vi "Turbo Process Mngr.vi"(0 "State In":T1, 1 "Mngr Action":T12, 2 "FP":T11, 7 "Cartridges":T5, 9 "Manual Input":dbl format="%#_13g", 11 "error in (no error)":errorcluster, 12 "Config":T2={"Syringe size"=0, "Syringe address"=0, "# of ports"=0, "Init String"="Z0N1R", "Full Stroke (cnts)"=0, "Model"=enum."XC", "TW Position"=0.0, "Load Position"=0.0, "Bottom Position"=0.0, "Station ID"="", "Default Protocol"=path "", "Dry Time(s)"=0.0, "Python Version"="", "NFC SN Array"=["21121521200223", "21121521200186", "21121521200213", "52541737200062"], "Timing"={"Checking pres and leak"=0.0, "Priming input lines"=0.0, "Rinsing syringe"=0.0, "Filling well X w/ X"=0.0, "Drain well X"=0.0, "Clearing wells and lines"=0.0, "Draining wells"=0.0, "Rinsing all wells"=0.0, "Testing for leaks/clogs"=0.0, "Rinsing wells"=0.0}, "Pressure Specs"={"Pressure max"=0.0, "Pressure min"=0.0, "Decay delta"=0.0, "Pressure time"=0.0, "Conf. R"=0.0, "LeakRateMax"=0.0}}) -> (15 "error out":errorcluster)   [LabVIEW 2020]
uses:
  Process Mngr.ctl
  Main Refs.ctl
  Wash Step.ctl
  Results.ctl
  Vacuum Test.ctl
  Pressure Output.ctl
  Process Turbo.ctl
  Cartridge #.ctl
  Hardware/Tecan/Pump Config.ctl
  Timing Specs.ctl
  Vacuum Specs.ctl
  status update.ctl
  Cartridge Mngr.ctl
  Time elapsed.ctl
  Hardware/DAQ Mngr.ctl
  Hardware/Mot Stage Mngr.ctl
  Update Single Cart.ctl
  Lib/Time/Bottles.ctl
  Hardware/16CH Denkovi Mngr.ctl
  Hardware/Tricon Mngr.ctl
  Hardware/Tecan/Pump Control.ctl
  Pump Port.ctl
  Hardware/Tecan/Velocity Units.ctl
  Main Globals.vi
  Lib/Utilities.lvlib
panel:
  out "State Out":T1
  out "Wash Time(s) 2":dbl
  out "Wash Time(s)":dbl
  out "Reports":T6[](array[typedef])
  in  "Pressure Specs":T9
  out "Wash Array":T10[](array[typedef]) {"# of Rinses" max=10}
  # "Tecan Pump"
  # "Pressure"
  # "General"
  # "Timing"
  # "Protocol"
  # "Zaber"
  # "NFC Reader 1"
  # "NFC  Reader 2"
  # "NFC Reader 3"
  # "NFC Reader 4"
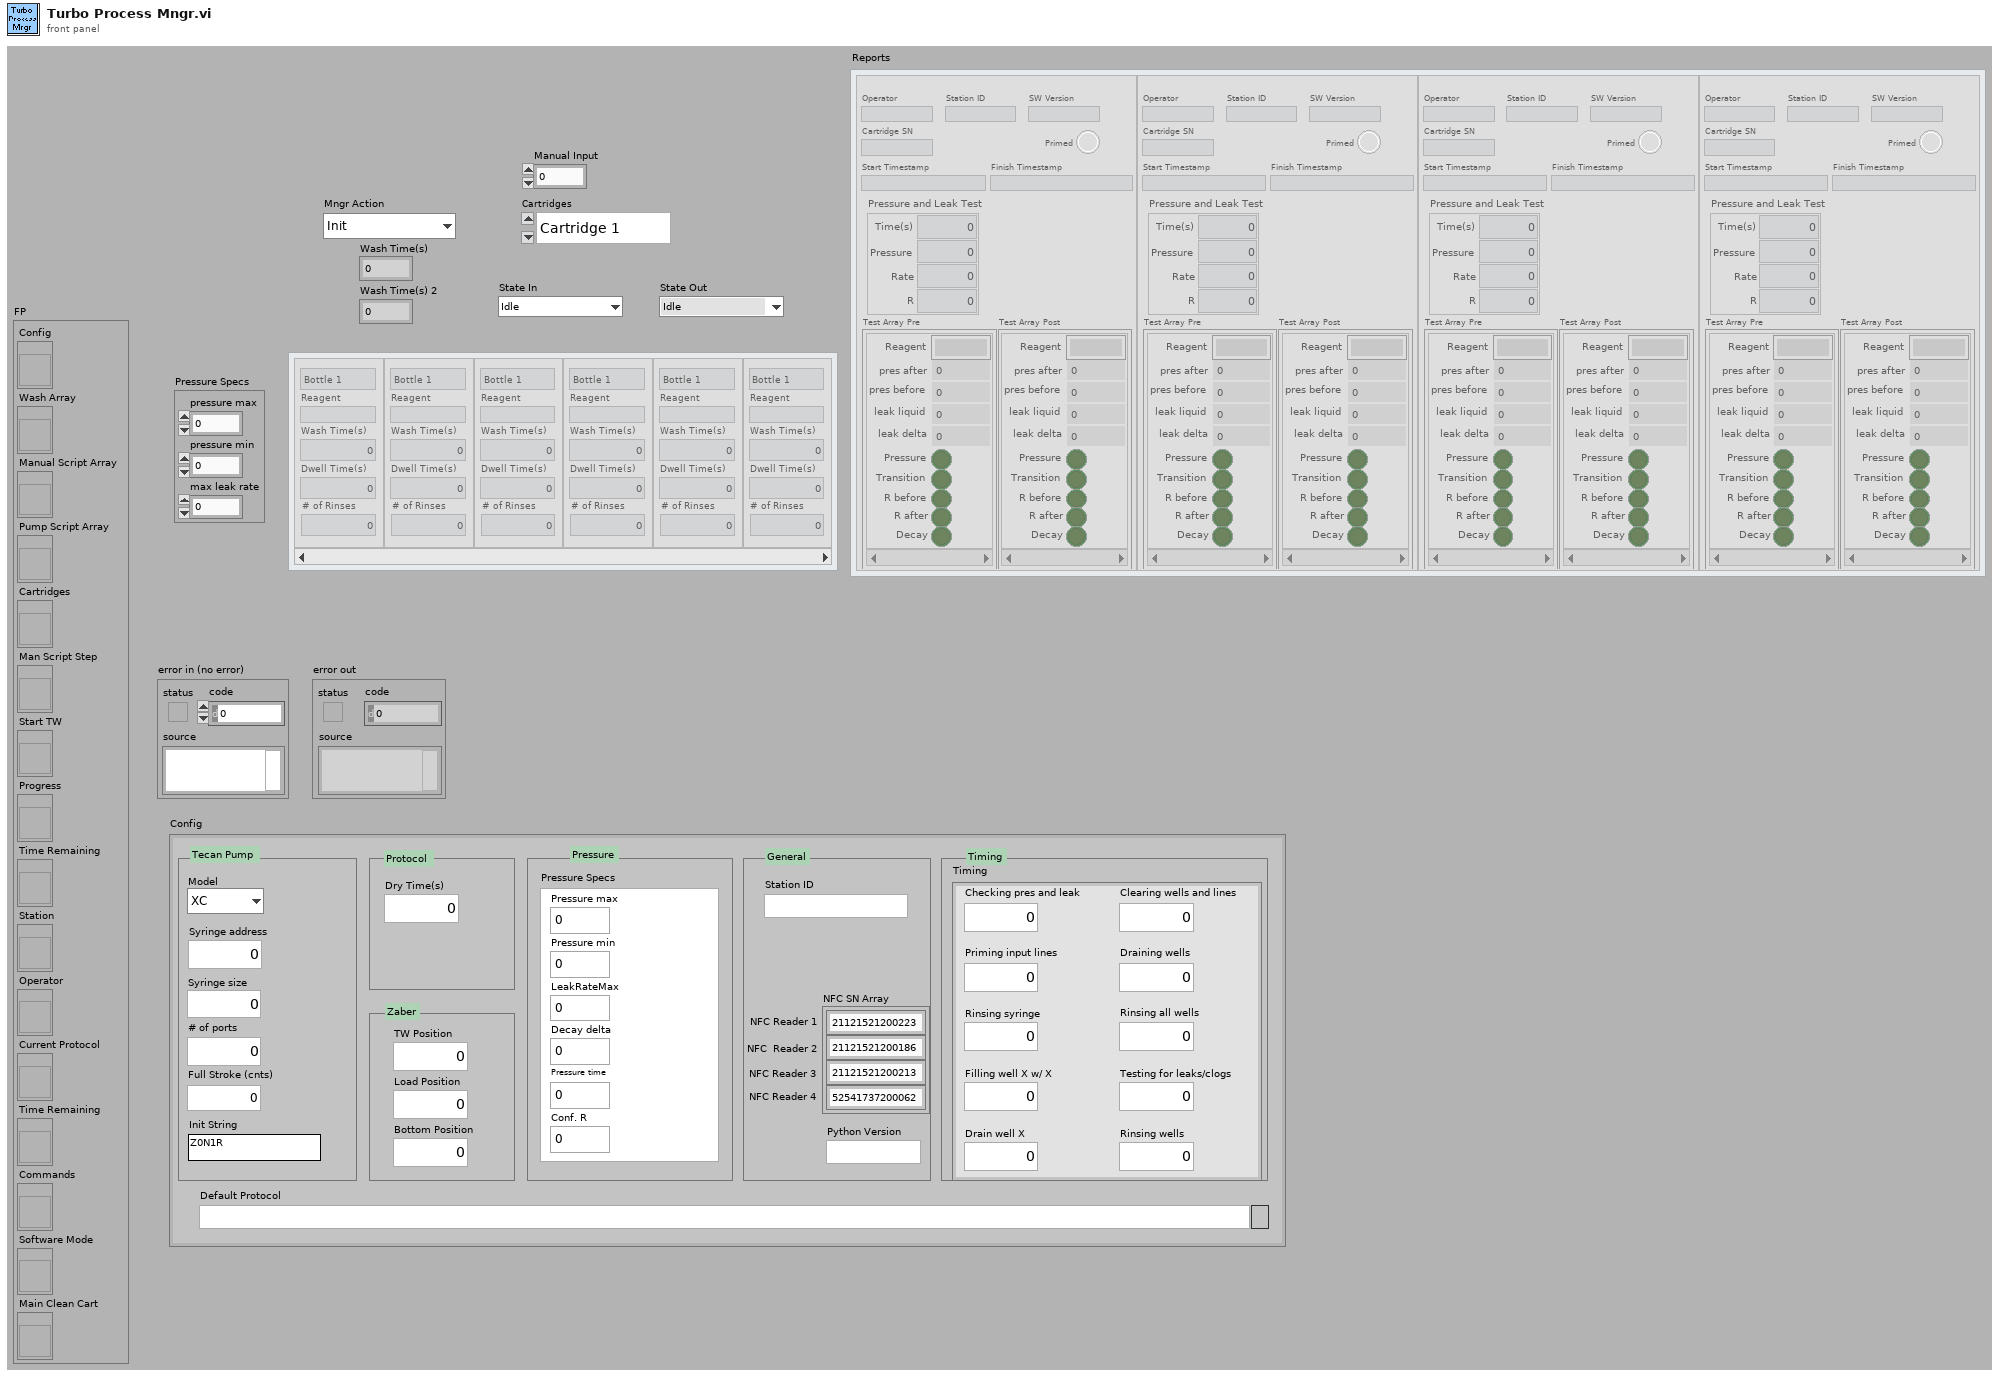
[diagram p1: front panel]
types:
  T1 = typedef "Process Turbo.ctl" = enum16{"Idle", "Init", "Check for SN", "Start TW", "SystemLeakTest", "Prime System", "Rinse Wells", "Fill Wells", "High Vac On", "Pressure&Vac Load", "Trap Vac", "PrePresTest", "Apply Pressure", "PostPresTest", "Drain&Rinse", "Dry", "Report", "Finish", "Abort", "Error", "-rinse wells", "-check cartridge", "-clean cartridge", "-drain all", "-fill well"}
  T2 = typedef "Pump Config.ctl" = cluster{"Syringe size":u32, "Syringe address":u32, "# of ports":u32, "Init String":string, "Full Stroke (cnts)":i32, "Model":enum16{"XC", "Centris"}, "TW Position":dbl, "Load Position":dbl, "Bottom Position":dbl, "Station ID":string, "Default Protocol":path, "Dry Time(s)":dbl, "Python Version":string, "NFC SN Array":string[], "Timing":T3, "Pressure Specs":T4}
  T3 = typedef "Timing Specs.ctl" = cluster{"Checking pres and leak":dbl, "Priming input lines":dbl, "Rinsing syringe":dbl, "Filling well X w/ X":dbl, "Drain well X":dbl, "Clearing wells and lines":dbl, "Draining wells":dbl, "Rinsing all wells":dbl, "Testing for leaks/clogs":dbl, "Rinsing wells":dbl}
  T4 = typedef "Vacuum Specs.ctl" = cluster{"Pressure max":dbl, "Pressure min":dbl, "Decay delta":dbl, "Pressure time":dbl, "Conf. R":dbl, "LeakRateMax":dbl}
  T5 = typedef "Cartridge #.ctl" = enum16{"Cartridge 1", "Cartridge 2", "Cartridge 3", "Cartridge 4"}
  T6 = typedef "Results.ctl" = cluster{"Operator":string, "Station ID":string, "SW Version":string, "Cartridge SN":string, "Primed":bool, "Start Timestamp":string, "Finish Timestamp":string, "Test Array Pre":T7[], "Test Array Post":T7[], "Pressure and Leak Test":T8}
  T7 = typedef "Vacuum Test.ctl" = cluster{"pres after":dbl, "pres before":dbl, "leak liquid":dbl, "leak delta":dbl, "Transition":bool, "Pressure":bool, "R before":bool, "R after":bool, "Reagent":string, "Decay":bool}
  T8 = typedef "Pressure Output.ctl" = cluster{"Time(s)":dbl, "Pressure":dbl, "Rate":dbl, "R":dbl}
  T9 = cluster{"pressure max":dbl, "pressure min":dbl, "max leak rate":dbl}
  T10 = typedef "Wash Step.ctl" = cluster{"Reagent":string, "Bottle":enum16{"Bottle 1", "Bottle 2", "Bottle 3", "Bottle 4"}, "Wash Time(s)":dbl, "Dwell Time(s)":dbl, "# of Rinses":i16}
  T11 = typedef "Main Refs.ctl" = cluster{"Config":refnum<vi>, "Wash Array":refnum<vi>, "Manual Script Array":refnum<vi>, "Pump Script Array":refnum<vi>, "Cartridges":refnum<vi>, "Man Script Step":refnum<vi>, "Start TW":refnum<vi>, "Progress":refnum<vi>, "Time Remaining":refnum<vi>, "Station":refnum<vi>, "Operator":refnum<vi>, "Current Protocol":refnum<vi>, "Time Remaining":refnum<vi>, "Commands":refnum<vi>, "Software Mode":refnum<vi>, "Main Clean Cart":refnum<vi>}
  T12 = typedef "Process Mngr.ctl" = enum16{"Init", "Run Step", "Update"}
  T13 = enum8{"Enabled", "Disabled", "Disabled and Grayed Out"}
  T14 = typedef "status update.ctl" = enum16{"Cartridge", "Main Status", "Reagent"}
  T15 = typedef "Cartridge Mngr.ctl" = enum16{"Init", "Update", "Detect", "Lock", "Read SN", "Unlock", "Error"}
  T16 = enum16{"Init Pressure", "Init Vacuum", "Save Pressure", "Save Vacuum", "Close"}
  T17 = typedef "DAQ Mngr.ctl" = enum16{"Init", "Read Pressure", "Read Vacuum", "Analyze Pres&Vac", "Analyze Vacuum", "Read Cartridges", "Lock Cartridge", "Unlock Cartridge", "Read PS", "Pinch Valve Engage", "Pinch Valve Disengage", "Close"}
  T18 = typedef "Time elapsed.ctl" = enum16{"Start", "Update", "Read"}
  T19 = typedef "Mot Stage Mngr.ctl" = enum16{"Connect", "Init", "Status", "Send Cmd", "Current Pos", "Set Accel", "Set Max Vel", "Home", "Rel Move", "Abs Move", "Close"}
  T20 = typedef "Update Single Cart.ctl" = enum16{"Cart Status", "Cart Reagent"}
  T21 = typedef "Bottles.ctl" = enum16{"Bottle 1", "Bottle 2", "Bottle 3", "H2O", "Waste"}
  T22 = typedef "16CH Denkovi Mngr.ctl" = enum16{"Search", "Init", "Set Peristaltic", "Set Pressure", "Set Vacuum", "Set PresVac", "Pres Vent&Close", "Vac Vent&Close", "Pres ON", "Vac ON", "Set All Relays", "Set One Relay", "Read Relays", "Close"}
  T23 = typedef "Pump Control.ctl" = cluster{"Syringe Pos":u32, "Rate":dbl, "Volume":dbl, "Valve":T24, "Action":enum32{"Withdraw", "Dispense", "Stop"}, "Move Type":enum32{"Abs", "Rel"}, "Init":bool, "Empty Syr.":bool, "Full Fill":bool, "Units":T25}
  T24 = typedef "Pump Port.ctl" = enum16{"Bottle 1", "Bottle 2", "Bottle 3", "Bottle 4", "Waste", "Well 1", "Well 2", "Well 3", "Well 4", "Bottle X", "Well X"}
  T25 = typedef "Velocity Units.ctl" = enum16{"ul/s", "ul/min"}
  T26 = typedef "Tricon Mngr.ctl" = enum16{"Init COM", "Set Config", "Init Pump", "Home", "Cmd", "Start Pump", "Set Valve", "Dispense", "Withdraw", "Status", "Close"}
  T27 = typedef "Cartridges.ctl" = cluster{"Cartridge 1":T28, "Cartridge 2":T28, "Cartridge 3":T28, "Cartridge 4":T28, "Current Status":string}
  T28 = typedef "Cartridge Status.ctl" = cluster{"Serial Number":string, "Reagent":string, "Cart Status":string, "Inserted":bool, "Eject":bool}
  T29 = typedef "Vacuum Output.ctl" = cluster{"Time(s)":dbl, "Vacuum":dbl, "Rate":dbl, "R":dbl}
  T30 = enum16{"Bottle 1", "Bottle 2", "Bottle 3", "Bottle 4"}
  T31 = typedef "Commands.ctl" = cluster{"Drain All Wells":bool, "Rinse All Wells":bool, "Prime":bool, "Well #":T32, "Bottle #":T21, "Fill":bool, "Run State":bool, "State":T33, "Empty Lines":bool, "Clean&Dry Cartridge":bool, "Check for leaks":bool, "Cart Test Array":T7[], "Number of rinses":dbl}
  T32 = typedef "Wells.ctl" = enum16{"Well 1", "Well 2", "Well 3", "Well 4"}
  T33 = typedef "Process State.ctl" = enum16{"Idle", "Init", "Check for SN", "Start TW", "SystemLeakTest", "Prime System", "Rinse Wells", "Fill Wells", "PrePresTest", "Apply Pressure", "PostPresTest", "Drain&Rinse", "Dry", "Report", "Finish", "Abort", "Error", "-rinse wells", "-check cartridge", "-clean cartridge", "-drain all", "-fill well"}
  T34 = cluster{"negative limit switch":bool, "positive limit switch":bool, "home switch":bool, "position marker":bool, "device enable":bool, "quick stop":bool, "general purpose J":bool, "general purpose I":bool, "general purpose H":bool, "general purpose G":bool, "general purpose F":bool, "general purpose E":bool, "general purpose D":bool, "general purpose C":bool, "general purpose B":bool, "general purpose A":bool}
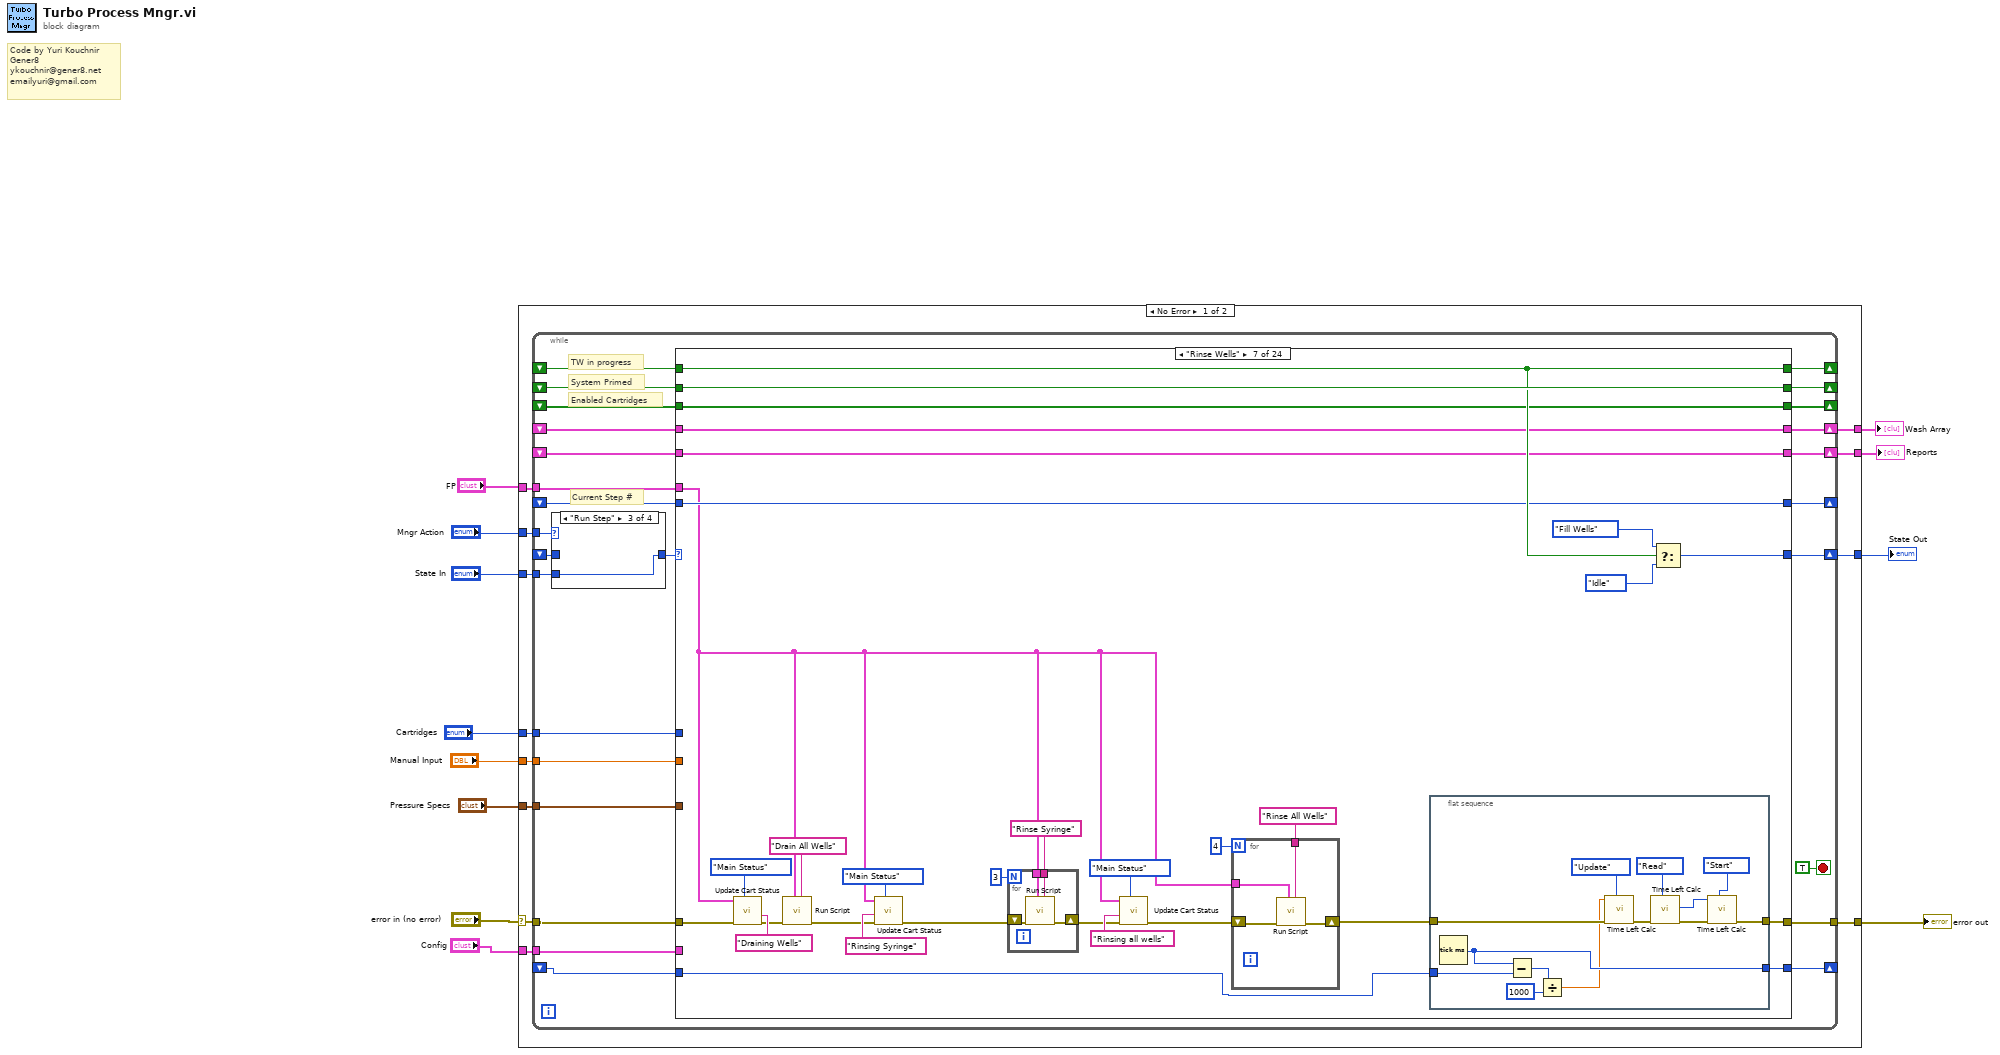
[diagram p0: block diagram]
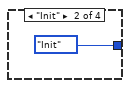
[diagram p3: hidden frame]
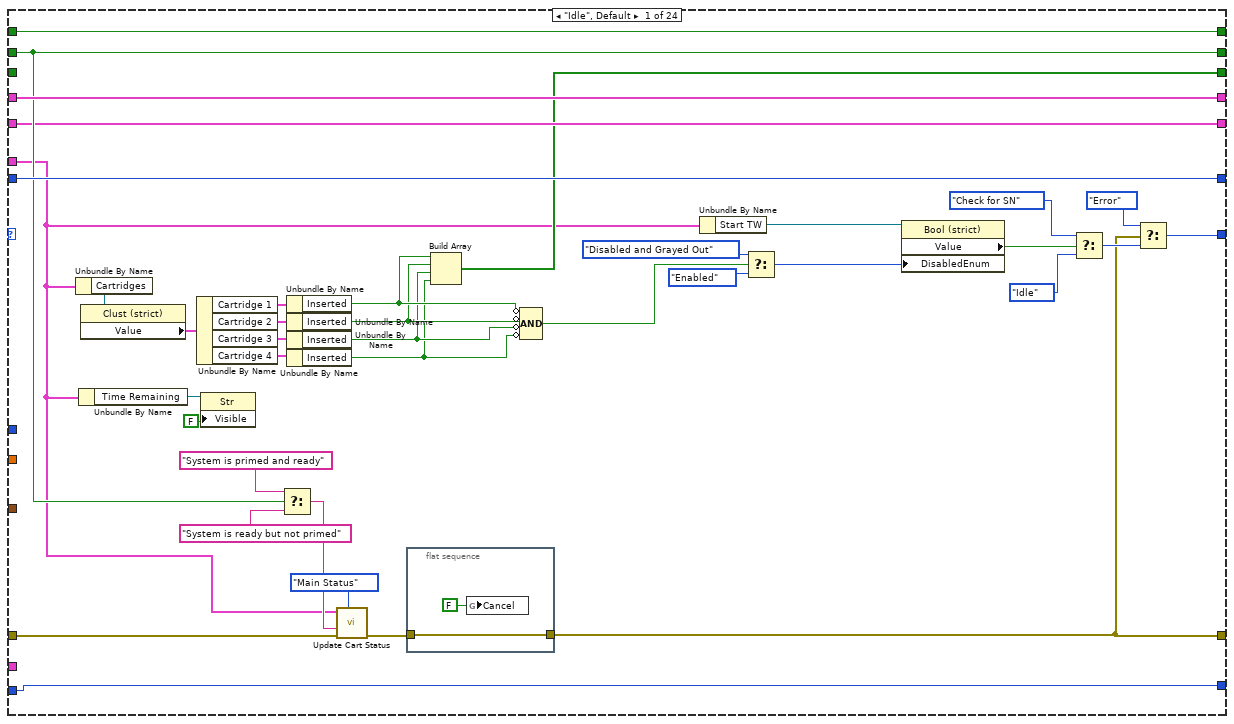
[diagram p5: hidden frame]
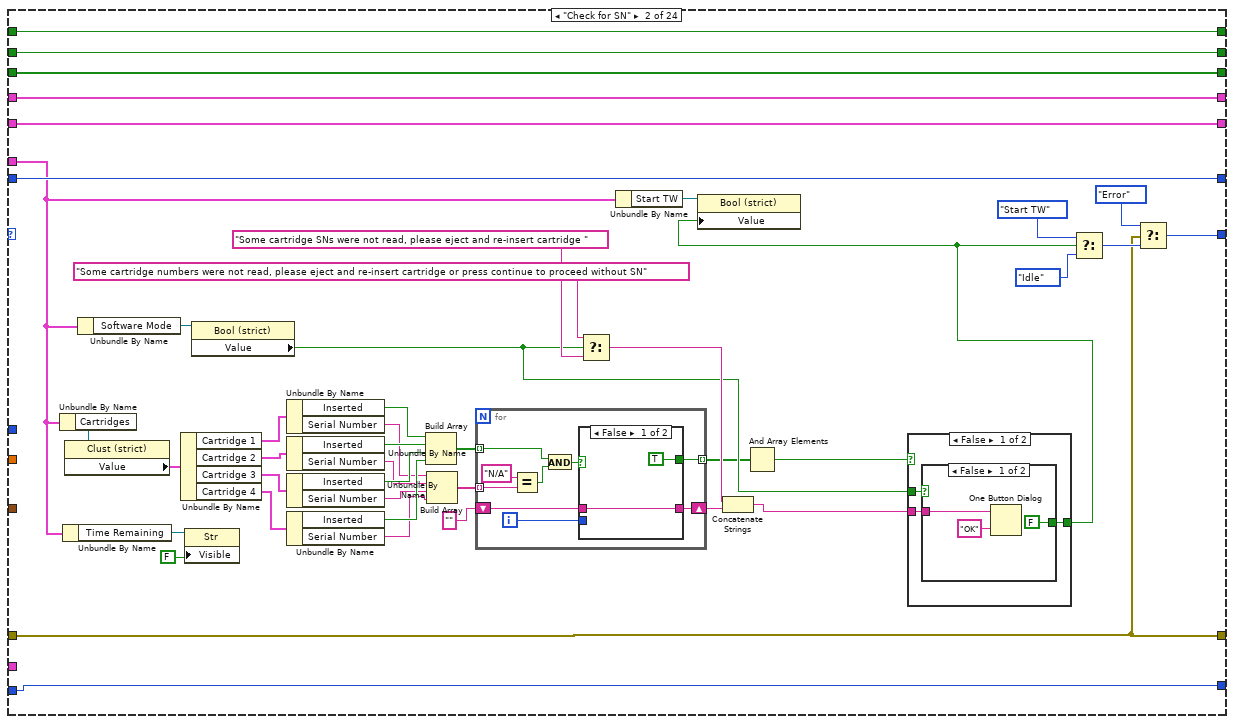
[diagram p6: hidden frame]
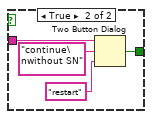
[diagram p7: hidden frame]
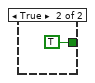
[diagram p8: hidden frame]
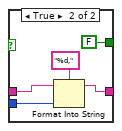
[diagram p9: hidden frame]
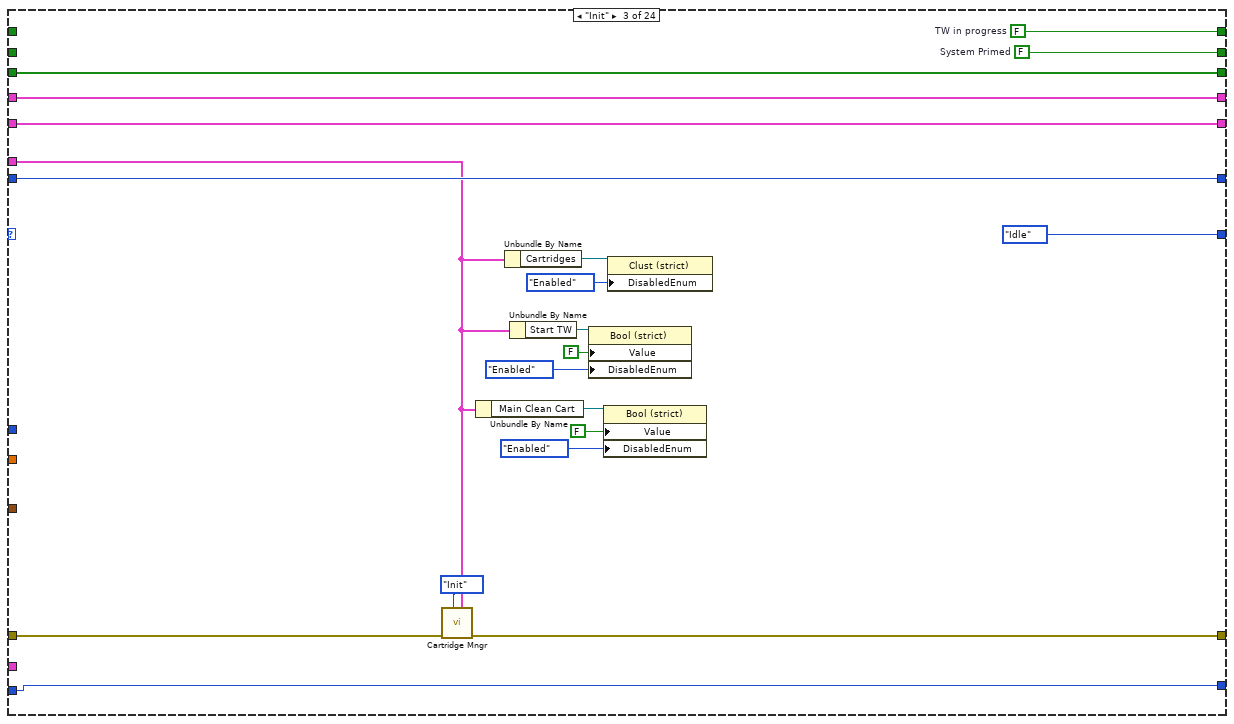
[diagram p10: hidden frame]
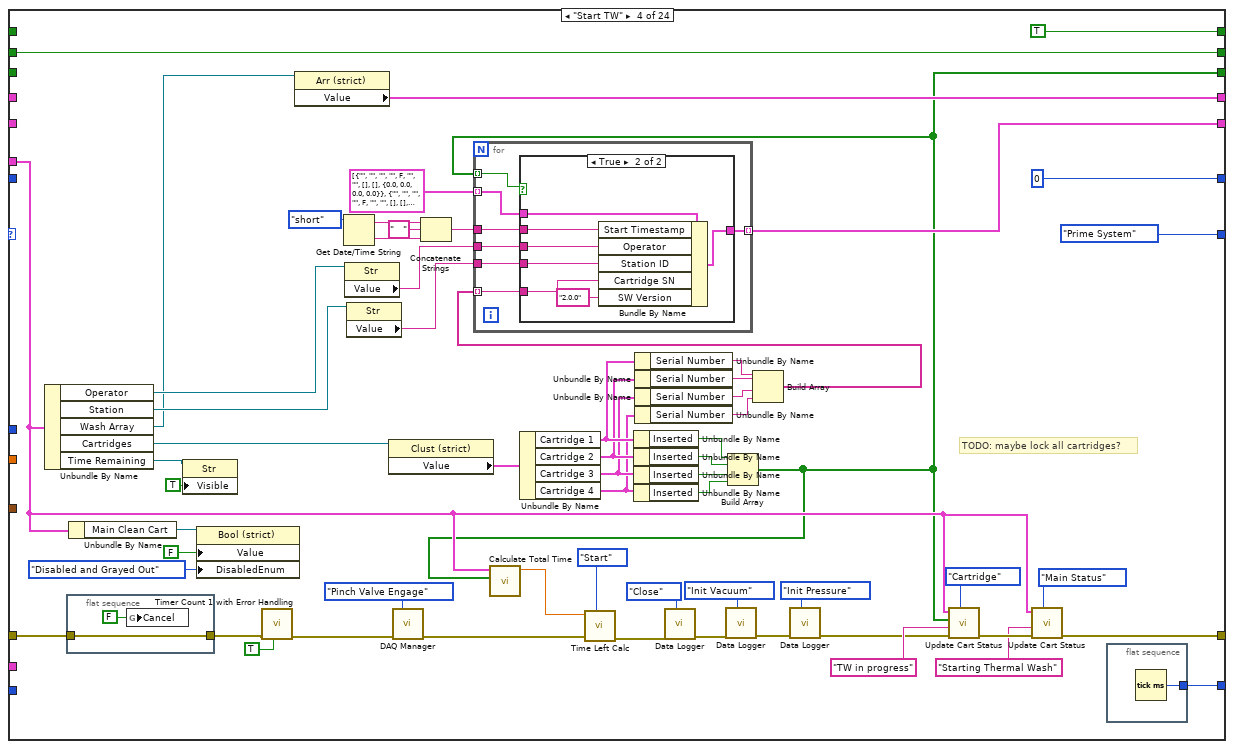
[diagram p11: hidden frame]
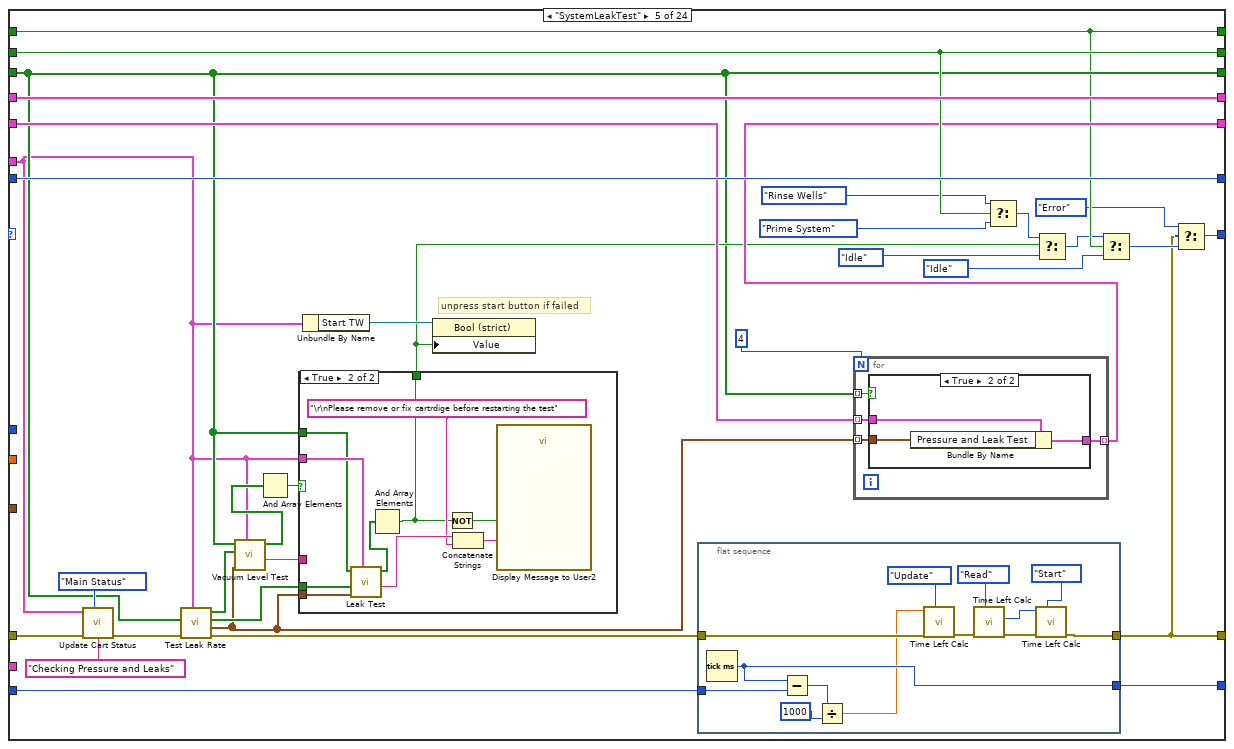
[diagram p13: hidden frame]
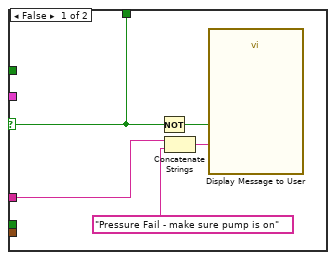
[diagram p14: hidden frame]
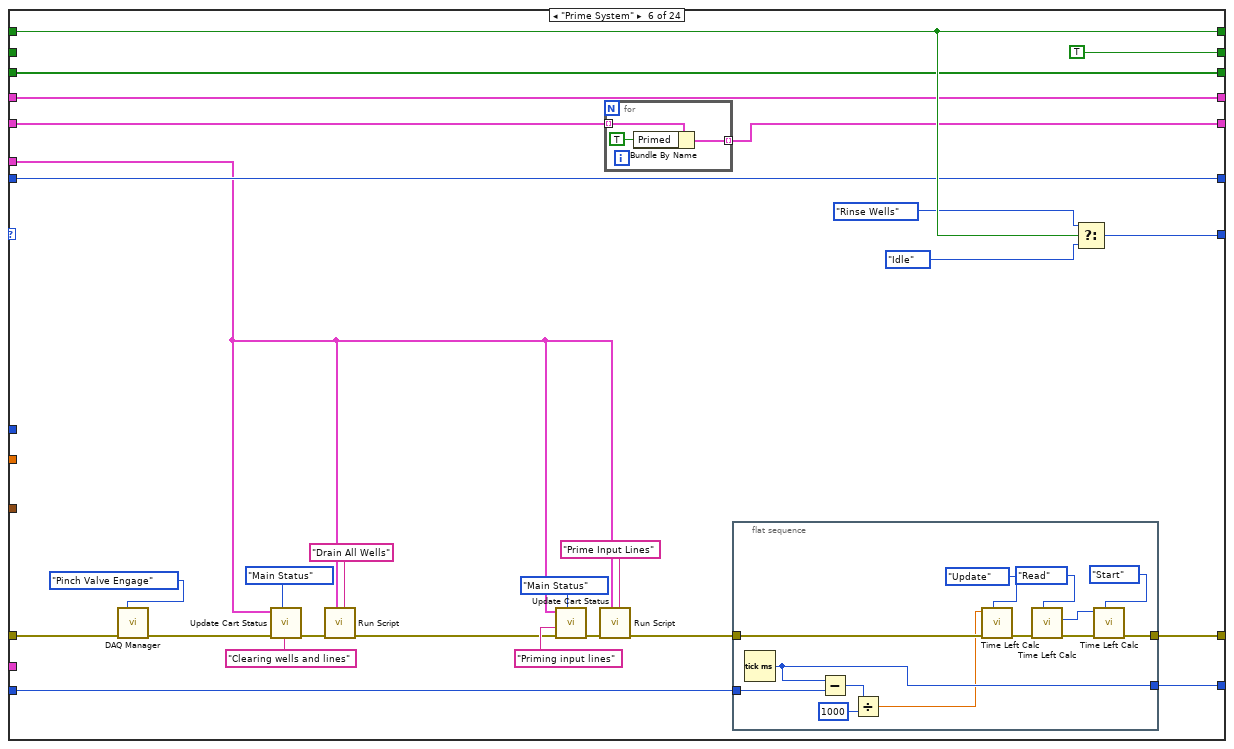
[diagram p16: hidden frame]
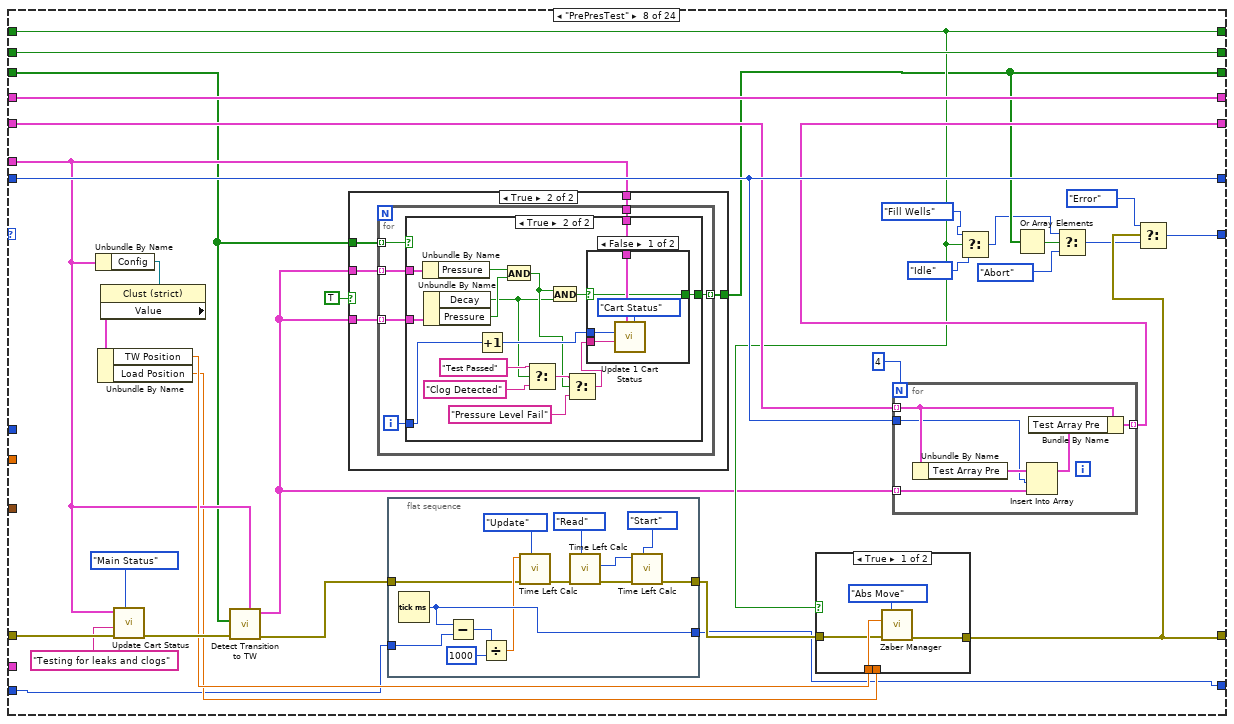
[diagram p17: hidden frame]
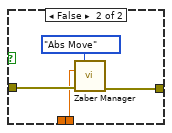
[diagram p18: hidden frame]
diagram:
  # "Code by Yuri Kouchnir\nGener8\nykouchnir@gener8.net\nemailyuri@gmail.com"
  n1 = case shown="No Error" "error in (no error)" {
    selector: "error in (no error)" -> [w24 w1427]
    tunnel: [w23 w1427] -> w11
    tunnel: "Mngr Action" -> [w22 _]
    tunnel: "FP" -> [w21 _]
    tunnel: "Pressure Specs" -> [w20 _]
    tunnel: [w19 _] -> w8
    tunnel: [w18 _] -> w6
    tunnel: "State In" -> [w17 _]
    tunnel: "Cartridges" -> [w16 _]
    tunnel: "Manual Input" -> [w15 _]
    tunnel: "Config" -> [w14 _]
    tunnel: [w13 _] -> w2
    frame No Error {
      n2 = while {
        tunnel: w24 -> [w50]
        tunnel: [w49] -> w23
        tunnel: w22 -> [w44]
        shift-right: [w48] -> w13
        shift-left: _ -> [w46]
        tunnel: w21 -> [w47]
        shift-right: [w43] -> _
        shift-left: _ -> [w42]
        shift-right: [w41] -> w19
        shift-left: _ -> [w40]
        shift-right: [w39] -> _
        shift-left: _ -> [w38]
        shift-right: [w37] -> _
        shift-left: _ -> [w36]
        shift-right: [w35] -> _
        shift-left: _ -> [w34]
        tunnel: w20 -> [w33]
        shift-right: [w32] -> w18
        shift-left: _ -> [w31]
        tunnel: w17 -> [w30]
        tunnel: w16 -> [w29]
        tunnel: w15 -> [w28]
        shift-right: [w27] -> _
        shift-left: _ -> [w26]
        tunnel: w14 -> [w25]
        stop <- TRUE stop-if-true
        # "Current Step #"
        # "Enabled Cartridges"
        # "System Primed"
        # "TW in progress"
        n3 = case shown="\"Run Step\"" w44 {
          tunnel: w46 -> [w52 _ _ w55]
          tunnel: [w52 Process_Turbo."Init" ("State In 2") w54 w55] -> w45
          tunnel: w30 -> [_ _ w54 _]
          frame Default {
          }
          frame "Init" {
          }
          frame "Run Step" {
          }
          frame "Update" {
          }
        }
        n4 = case shown="\"Rinse Wells\"" w45 {
          tunnel: w50 -> [w66 w107 w168 w215 w296 w337 w400 w458 w536 w617 w685 w753 w820 w901 w1017 w1065 w1100 w1118 w1180 w1198 w1233 w1256 w1315 w1388]
          tunnel: [w64 w107 w181 w236 w274 w346 w382 w442 w531 w608 w677 w744 w809 w893 w1005 w1064 w1093 w1120 w1172 w1190 w1225 w1250 w1303 w1371] -> w49
          tunnel: [w87 w134 Process_Turbo."Idle" ("State In 2") Process_Turbo."Prime System" ("State In 2") w295 w361 w408 w461 w546 w629 w697 w765 w823 w922 w1025 Process_Turbo."Idle" ("State In 2") Process_Turbo."Idle" ("State In 2") Process_Turbo."Finish" ("State In 2") Process_Turbo."Idle" ("State In 2") w1208 w1241 w1264 w1318 w1391] -> w48
          tunnel: w47 -> [w61 w109 w170 w198 w275 w348 w384 w449 w532 w606 w675 w742 w812 w902 w1009 w1067 w1084 w1116 w1163 w1191 w1236 w1259 w1286 w1376]
          tunnel: [w85 w133 w186 w213 w294 TRUE ("System Primed") w407 w462 w550 w632 w700 w768 w825 w924 w1034 w1079 w1110 w1130 w1185 w1209 w1244 w1267 w1306 w1378] -> w43
          tunnel: w42 -> [w85 w133 _ w213 w294 _ w407 w462 w550 w632 w700 w768 w825 w924 w1034 w1079 w1110 w1130 w1185 w1209 w1244 w1267 w1306 w1378]
          tunnel: [w91 w137 w182 w205 w298 w357 w403 w460 w541 w621 w689 w758 w822 w918 w1024 w1078 w1109 w1129 w1184 w1207 w1239 w1262 w1317 w1390] -> w41
          tunnel: w40 -> [w91 w137 w182 _ w298 w357 w403 w460 w541 w621 w689 w758 w822 w918 w1024 w1078 w1109 w1129 w1184 w1207 w1239 w1262 w1317 w1390]
          tunnel: [w93 w139 w185 TRUE ("TW in progress") w278 w360 w406 w447 w548 w631 w699 w767 w807 w897 w1020 w1077 FALSE ("TW in progress") w1128 FALSE ("TW in progress") w1195 w1243 w1266 w1311 w1384] -> w39
          tunnel: w38 -> [w93 w139 _ _ w278 w360 w406 w447 w548 w631 w699 w767 w807 w897 w1020 w1077 _ w1128 _ w1195 w1243 w1266 w1311 w1384]
          tunnel: [w92 w138 w183 0 w297 w358 w404 w454 w545 w626 w694 w763 w816 w919 w1021 w1076 w1108 w1127 w1183 w1194 w1240 w1263 w1312 w1385] -> w37
          tunnel: w36 -> [w92 w138 w183 _ w297 w358 w404 w454 w545 w626 w694 w763 w816 w920 w1021 w1076 w1108 w1127 w1183 w1194 w1240 w1263 w1312 w1385]
          tunnel: [w67 w119 w184 w197 w279 w359 w405 w436 w534 w614 w662 w750 w811 w907 w1008 w1075 w1107 w1114 w1181 w1189 w1237 w1260 w1270 w1366] -> w35
          tunnel: w34 -> [_ w119 w184 _ w279 w359 w405 w446 w534 w614 w662 w750 w798 w907 w1008 w1075 w1107 w1114 w1181 w1189 w1237 w1260 w1270 w1366]
          tunnel: w33 -> [_ _ _ _ _ _ _ _ _ w622 w690 w760 _ _ w1029 _ _ _ _ _ _ _ _ _]
          tunnel: [w81 w132 w174 w229 w287 w353 w386 w452 w539 w620 w688 w756 w814 w916 w1019 w1066 w1106 w1119 w1170 w1206 w1238 w1261 w1287 w1370] -> w32
          tunnel: w31 -> [w81 w132 w174 _ w289 w354 w386 w453 w539 w620 w688 w756 w815 w916 w1019 w1066 w1106 w1121 w1170 w1206 w1238 w1261 w1287 w1370]
          tunnel: w29 -> [_ _ _ _ _ _ _ _ _ _ _ _ _ _ _ _ _ _ _ _ _ _ _ _]
          tunnel: w28 -> [_ _ _ _ _ _ _ _ _ _ _ _ _ _ _ _ _ _ _ w1193 _ _ _ _]
          tunnel: [w59 w99 w169 w196 w271 w344 w380 w439 w530 w607 w676 w743 w800 w892 w1003 w1063 w1092 w1113 w1162 w1188 w1224 w1248 w1285 w1364] -> w27
          tunnel: w26 -> [w59 w99 w169 _ w273 w347 w383 w438 w528 _ _ _ w799 w891 _ w1063 w1092 w1113 w1162 w1188 w1224 w1248 w1285 w1364]
          tunnel: w25 -> [_ _ _ _ _ _ _ _ _ _ _ _ _ _ _ _ w1090 _ _ _ _ _ _ _]
          frame "Idle", Default {
            n5 = Unbundle By Name(w61) -> ("Cartridges"=w76:refnum<vi>)
            n6 = Unbundle By Name(w61) -> ("Time Remaining"=w63:refnum<vi>)
            n7 = property class="Clust (strict)"(reference=w76) -> ("Value"=w80:T27)  [unwired: 1 in, 2 out]
            n8 = Unbundle By Name(w80) -> ("Cartridge 1"=w75:T28, "Cartridge 2"=w79:T28, "Cartridge 3"=w78:T28, "Cartridge 4"=w77:T28)
            n9 = property class="Str"(reference=w63, "Visible"=FALSE) -> ()  [unwired: 1 in, 2 out]
            n10 = Select(t="System is primed and ready" ("Reagent"), s=w85, f="System is ready but not primed" ("Reagent")) -> (s? t:f=w82:string)
            n11 = Unbundle By Name(w75) -> ("Inserted"=w71:bool)
            n12 = Unbundle By Name(w79) -> ("Inserted"=w70:bool)
            n13 = Unbundle By Name(w78) -> ("Inserted"=w69:bool)
            n14 = Unbundle By Name(w77) -> ("Inserted"=w68:bool)
            n15 = call "Update Cart Status.vi"("Selection"=status_update."Main Status", "error in (no error)"=w66, "String"=w82, "FP"=w61) -> ("error out"=w65:errorcluster)  [unwired: 7 in]
            n16 = flat-sequence {
              tunnel: w65 -> [w95]
              tunnel: [w95] -> w64
              frame #0 {
                n17 = global write "Main Globals.vi" "Cancel"(FALSE ("Cancel")) -> ()
              }
            }
            n18 = Build Array(w71, w70, w69, w68) -> (w67:bool[])
            n19 = Compound Arithmetic op=AND(invert w71, invert w70, invert w69, invert w68) -> (w60:bool)
            n20 = Unbundle By Name(w61) -> ("Start TW"=w90:refnum<vi>)
            n21 = Select(t=T13."Disabled and Grayed Out" ("Disabled"), s=w60, f=T13."Enabled" ("Disabled")) -> (s? t:f=w72:T13)
            n22 = property class="Bool (strict)"(reference=w90, "DisabledEnum"=w72) -> ("Value"=w89:bool)  [unwired: 1 in, 2 out]
            n23 = Select(t=Process_Turbo."Check for SN" ("State In 2"), s=w89, f=Process_Turbo."Idle") -> (s? t:f=w88:T1)
            n24 = Select(t=Process_Turbo."Error", s=w64, f=w88) -> (s? t:f=w87:T1)
          }
          frame "Check for SN" {
            n25 = Unbundle By Name(w109) -> ("Cartridges"=w127:refnum<vi>)
            n26 = Unbundle By Name(w109) -> ("Time Remaining"=w121:refnum<vi>)
            n27 = property class="Clust (strict)"(reference=w127) -> ("Value"=w131:T27)  [unwired: 1 in, 2 out]
            n28 = Unbundle By Name(w109) -> ("Software Mode"=w108:refnum<vi>)
            n29 = Unbundle By Name(w131) -> ("Cartridge 1"=w126:T28, "Cartridge 2"=w130:T28, "Cartridge 3"=w129:T28, "Cartridge 4"=w128:T28)
            n30 = property class="Str"(reference=w121, "Visible"=FALSE) -> ()  [unwired: 1 in, 2 out]
            n31 = property class="Bool (strict)"(reference=w108) -> ("Value"=w103:bool)  [unwired: 1 in, 2 out]
            n32 = Unbundle By Name(w126) -> ("Inserted"=w125:bool, "Serial Number"=w118:string)
            n33 = Unbundle By Name(w130) -> ("Inserted"=w124:bool, "Serial Number"=w117:string)
            n34 = Unbundle By Name(w129) -> ("Inserted"=w123:bool, "Serial Number"=w116:string)
            n35 = Unbundle By Name(w128) -> ("Inserted"=w122:bool, "Serial Number"=w115:string)
            n36 = Build Array(w125, w124, w123, w122) -> (w114:bool[])
            n37 = Build Array(w118, w117, w116, w115) -> (w113:string[])
            n38 = for {
              tunnel: w114 -> [w154] mode=indexing
              tunnel: w113 -> [w157] mode=indexing
              shift-right: [w152] -> w110
              shift-left: "" ("Serial Number") -> [w158]
              tunnel: [w151] -> w102 mode=indexing
              i -> [w159]
              n39 = Equal?(x="N/A", y=w157) -> (x = y?=w155:bool)
              n40 = And(x=w154, y=w155) -> (x .and. y?=w153:bool)
              n41 = case shown="False" w153 {
                tunnel: w159 -> [_ w166]
                tunnel: w158 -> [w161 w165]
                tunnel: [w161 w164] -> w152
                tunnel: [TRUE FALSE] -> w151
                frame False {
                }
                frame True {
                  n42 = Format Into String(format string="%d,", initial string=w165, w166) -> (resulting string=w164:string)  [unwired: 1 in, 1 out]
                }
              }
            }
            n43 = Select(t="Some cartridge numbers were not read, please eject and re-insert cartridge or press continue to proceed without SN" ("message"), s=w103, f="Some cartridge SNs were not read, please eject and re-insert cartridge " ("message")) -> (s? t:f=w104:string)
            n44 = Unbundle By Name(w109) -> ("Start TW"=w136:refnum<vi>)
            n45 = Concatenate Strings(w104, w110) -> (w111:string)
            n46 = And Array Elements(Boolean array=w102) -> (logical AND=w101:bool)
            n47 = case shown="False" w101 {
              tunnel: w111 -> [w142 _]
              tunnel: w103 -> [w141 _]
              tunnel: [w140 TRUE ("T button?")] -> w100
              frame False {
                n48 = case shown="False" w141 {
                  tunnel: w142 -> [w144 w149]
                  tunnel: [FALSE ("T button?") w146] -> w140
                  frame False {
                    n49 = One Button Dialog(message=w144, button name ("OK")="OK") -> ()  [unwired: 1 out]
                  }
                  frame True {
                    n50 = Two Button Dialog(message=w149, 1:"restart" ("T button name (\"OK\")"), 2:"continue\nwithout SN" ("T button name (\"OK\")")) -> (T button?=w146:bool)
                  }
                }
              }
              frame True {
              }
            }
            n51 = property class="Bool (strict)"(reference=w136, "Value"=w100) -> ()  [unwired: 1 in, 2 out]
            n52 = Select(t=Process_Turbo."Start TW" ("State In 2"), s=w100, f=Process_Turbo."Idle" ("State In 2")) -> (s? t:f=w135:T1)
            n53 = Select(t=Process_Turbo."Error" ("State In 2"), s=w107, f=w135) -> (s? t:f=w134:T1)
          }
          frame "Init" {
            w185 = FALSE  # TW in progress
            w186 = FALSE  # System Primed
            n54 = call "Cartridge Mngr.vi"("Main References"=w170, "Mngr Action"=Cartridge_Mngr."Init", "error in (no error)"=w168) -> ("error out"=w181:errorcluster)  [unwired: 6 in, 2 out]
            n55 = Unbundle By Name(w170) -> ("Main Clean Cart"=w171:refnum<vi>)
            n56 = Unbundle By Name(w170) -> ("Cartridges"=w179:refnum<vi>)
            n57 = Unbundle By Name(w170) -> ("Start TW"=w177:refnum<vi>)
            n58 = property class="Bool (strict)"(reference=w177, "Value"=FALSE, "DisabledEnum"=T13."Enabled" ("Disabled")) -> ()  [unwired: 1 in, 2 out]
            n59 = property class="Bool (strict)"(reference=w171, "Value"=FALSE, "DisabledEnum"=T13."Enabled" ("Disabled")) -> ()  [unwired: 1 in, 2 out]
            n60 = property class="Clust (strict)"(reference=w179, "DisabledEnum"=T13."Enabled" ("Disabled")) -> ()  [unwired: 1 in, 2 out]
          }
          frame "Start TW" {
            # "TODO: maybe lock all cartridges?"
            n61 = Unbundle By Name(w198) -> ("Operator"=w219:refnum<vi>, "Station"=w217:refnum<vi>, "Wash Array"=w209:refnum<vi>, "Cartridges"=w214:refnum<vi>, "Time Remaining"=w203:refnum<vi>)
            n62 = flat-sequence {
              tunnel: w215 -> [w250]
              tunnel: [w250] -> w211
              frame #0 {
                n63 = global write "Main Globals.vi" "Cancel"(FALSE ("Cancel")) -> ()
              }
            }
            n64 = Unbundle By Name(w198) -> ("Main Clean Cart"=w199:refnum<vi>)
            n65 = property class="Str"(reference=w203, "Visible"=TRUE) -> ()  [unwired: 1 in, 2 out]
            n66 = property class="Bool (strict)"(reference=w199, "Value"=FALSE, "DisabledEnum"=T13."Disabled and Grayed Out" ("Disabled")) -> ()  [unwired: 1 in, 2 out]
            n67 = call "Timer Count 1 with Error Handling.vi"("Reset"=TRUE, "error in (no error)"=w211) -> ("error out"=w194:errorcluster)  [unwired: 6 in, 3 out]
            n68 = property class="Arr (strict)"(reference=w209) -> ("Value"=w205:T10[])  [unwired: 1 in, 2 out]
            n69 = Get Date/Time String(date format (0)=enum16{"short", "long", "abbreviated"}."short") -> (date string=w233:string, time string=w232:string)  [unwired: 2 in]
            n70 = property class="Str"(reference=w219) -> ("Value"=w218:string)  [unwired: 1 in, 2 out]
            n71 = property class="Str"(reference=w217) -> ("Value"=w216:string)  [unwired: 1 in, 2 out]
            n72 = property class="Clust (strict)"(reference=w214) -> ("Value"=w212:T27)  [unwired: 1 in, 2 out]
            n73 = call "DAQ Manager.vi"("DAQ Mngr Action"=DAQ_Mngr."Pinch Valve Engage", "error in (no error)"=w194) -> ("error out"=w193:errorcluster)  [unwired: 6 in, 7 out]
            n74 = Concatenate Strings(w233, "   " ("string"), w232) -> (w230:string)
            n75 = Unbundle By Name(w212) -> ("Cartridge 1"=w228:T28, "Cartridge 2"=w227:T28, "Cartridge 3"=w226:T28, "Cartridge 4"=w225:T28)
            n76 = Unbundle By Name(w228) -> ("Inserted"=w245:bool)
            n77 = Unbundle By Name(w227) -> ("Inserted"=w244:bool)
            n78 = Unbundle By Name(w226) -> ("Inserted"=w243:bool)
            n79 = Unbundle By Name(w225) -> ("Inserted"=w242:bool)
            n80 = Unbundle By Name(w228) -> ("Serial Number"=w224:string)
            n81 = Unbundle By Name(w227) -> ("Serial Number"=w223:string)
            n82 = Unbundle By Name(w226) -> ("Serial Number"=w222:string)
            n83 = Unbundle By Name(w225) -> ("Serial Number"=w221:string)
            n84 = Build Array(w245, w244, w243, w242) -> (w197:bool[])
            n85 = call "Calculate Total Time.vi"("Boolean array"=w197, "FP"=w198) -> ("Total Time(s)"=w204:dbl)  [unwired: 9 in]
            n86 = call "Time Left Calc.vi"("Enum"=Time_elapsed."Start", "error in (no error)"=w193, "Time"=w204) -> ("error out"=w207:errorcluster)  [unwired: 6 in, 2 out]
            n87 = call "Data Logger.vi"("Action"=T16."Close", "error in"=w207) -> ("error out"=w208:errorcluster)  [unwired: 9 in]
            n88 = call "Data Logger.vi"("Action"=T16."Init Vacuum", "error in"=w208) -> ("error out"=w192:errorcluster)  [unwired: 9 in]
            n89 = Build Array(w224, w223, w222, w221) -> (w220:string[])
            n90 = for {
              tunnel: T6[] [{"Operator"="", "Station ID"="", "SW Version"="", "Cartridge SN"="", "Primed"=FALSE, "Start Timestamp"="", "Finish Timestamp"="", "Test Array Pre"=[], "Test Array Post"=[], "Pressure and Leak Test"={"Time(s)"=0.0, "Pressure"=0.0, "Rate"=0.0, "R"=0.0}}, {"Operator"="", "Station ID"="", "SW Version"="", "Cartridge SN"="", "Primed"=FALSE, "Start Timestamp"="", "Finish Timestamp"="", "Test Array Pre"=[], "Test Array Post"=[], "Pressure and Leak Test"={"Time(s)"=0.0, "Pressure"=0.0, "Rate"=0.0, "R"=0.0}}, {"Operator"="", "Station ID"="", "SW Version"="", "Cartridge SN"="", "Primed"=FALSE, "Start Timestamp"="", "Finish Timestamp"="", "Test Array Pre"=[], "Test Array Post"=[], "Pressure and Leak Test"={"Time(s)"=0.0, "Pressure"=0.0, "Rate"=0.0, "R"=0.0}}, {"Operator"="", "Station ID"="", "SW Version"="", "Cartridge SN"="", "Primed"=FALSE, "Start Timestamp"="", "Finish Timestamp"="", "Test Array Pre"=[], "Test Array Post"=[], "Pressure and Leak Test"={"Time(s)"=0.0, "Pressure"=0.0, "Rate"=0.0, "R"=0.0}}] ("Reports") -> [w257] mode=indexing
              tunnel: w230 -> [w256]
              tunnel: [w255] -> w229 mode=indexing
              tunnel: w197 -> [w254] mode=indexing
              tunnel: w220 -> [w253] mode=indexing
              tunnel: w218 -> [w252]
              tunnel: w216 -> [w251]
              n91 = case shown="True" w254 {
                tunnel: w257 -> [w258 w265]
                tunnel: w256 -> [_ w264]
                tunnel: [w258 w263] -> w255
                tunnel: w253 -> [_ w262]
                tunnel: w252 -> [_ w261]
                tunnel: w251 -> [_ w260]
                frame False {
                }
                frame True {
                  n92 = Bundle By Name(cluster=w265, "Start Timestamp"=w264, "Operator"=w261, "Station ID"=w260, "Cartridge SN"=w262, "SW Version"="2.0.0") -> (w263:T6)
                }
              }
            }
            n93 = call "Data Logger.vi"("Action"=T16."Init Pressure", "error in"=w192) -> ("error out"=w191:errorcluster)  [unwired: 9 in]
            n94 = call "Update Cart Status.vi"("Selection"=status_update."Cartridge", "error in (no error)"=w191, "String"="TW in progress" ("Reagent"), "Array"=w197, "FP"=w198) -> ("error out"=w240:errorcluster)  [unwired: 6 in]
            n95 = call "Update Cart Status.vi"("Selection"=status_update."Main Status", "error in (no error)"=w240, "String"="Starting Thermal Wash" ("Reagent"), "FP"=w198) -> ("error out"=w236:errorcluster)  [unwired: 7 in]
            n96 = flat-sequence {
              tunnel: [w248] -> w196
              frame #0 {
                n97 = Tick Count (ms)() -> (millisecond timer value=w248:u32)
              }
            }
          }
          frame "SystemLeakTest" {
            # "unpress start button if failed"
            n98 = call "Update Cart Status.vi"("Selection"=status_update."Main Status", "String"="Checking Pressure and Leaks" ("Reagent"), "FP"=w275) -> ()  [unwired: 8 in, 1 out]
            n99 = call "Test Leak Rate.vi"("Main References"=w275, "error in (no error)"=w296, "Cart Array"=w279) -> ("error out"=w272:errorcluster, "Results"=w281:T29[], "RatePass"=w282:bool[], "Pres Pass"=w286:bool[])  [unwired: 5 in]
            n100 = call "Vacuum Level Test.vi"("FP"=w275, "Results"=w281, "Pres Pass"=w286, "Cart Array"=w279) -> ("Error String"=w284:string, "Pass/Fail Array"=w280:bool[])  [unwired: 6 in]
            n101 = And Array Elements(Boolean array=w280) -> (logical AND=w285:bool)
            n102 = case shown="True" w285 {
              selector: w285 -> [w312 _]
              tunnel: w284 -> [w314 _]
              tunnel: [w312 w319] -> w283
              tunnel: w282 -> [_ w326]
              tunnel: w275 -> [_ w325]
              tunnel: w281 -> [_ w324]
              tunnel: w279 -> [_ w318]
              frame False {
                n103 = Not(x=w312) -> (.not. x?=w316:bool)
                n104 = Concatenate Strings(w314, "Pressure Fail - make sure pump is on" ("string")) -> (w315:string)
                n105 = call "Display Message to User"("Enable"=w316, "Message"=w315) -> ()  [unwired: 8 in, 2 out]
              }
              frame True {
                n106 = call "Leak Test.vi"("FP"=w325, "Results"=w324, "RatePass"=w326, "Cart Array"=w318) -> ("Error String"=w323:string, "Pass/Fail Array"=w317:bool[])  [unwired: 6 in]
                n107 = And Array Elements(Boolean array=w317) -> (logical AND=w319:bool)
                n108 = Not(x=w319) -> (.not. x?=w322:bool)
                n109 = Concatenate Strings(w323, "\r\nPlease remove or fix cartrdige before restarting the test" ("string")) -> (w321:string)
                n110 = call "Display Message to User2"("Enable"=w322, "Message"=w321) -> ()  [unwired: 8 in, 2 out]
              }
            }
            n111 = Unbundle By Name(w275) -> ("Start TW"=w292:refnum<vi>)
            n112 = property class="Bool (strict)"(reference=w292, "Value"=w283) -> ()  [unwired: 1 in, 2 out]
            n113 = flat-sequence {
              tunnel: [w308] -> w274
              tunnel: w273 -> [w307]
              tunnel: w272 -> [w305]
              tunnel: [w302] -> w271
              frame #0 {
                n114 = Tick Count (ms)() -> (millisecond timer value=w302:u32)
                n115 = Subtract(x=w302, y=w307) -> (x-y=w299:u32)
                n116 = Divide(x=w299, y=u32 1000) -> (x/y=w301:dbl)
                n117 = call "Time Left Calc.vi"("Enum"=Time_elapsed."Update", "error in (no error)"=w305, "Time"=w301) -> ("error out"=w304:errorcluster)  [unwired: 6 in, 2 out]
                n118 = call "Time Left Calc.vi"("Enum"=Time_elapsed."Read", "error in (no error)"=w304) -> ("error out"=w310:errorcluster, "Time Left"=w309:u32)  [unwired: 7 in, 1 out]
                n119 = call "Time Left Calc.vi"("Enum"=Time_elapsed."Start", "error in (no error)"=w310, "Time"=w309) -> ("error out"=w308:errorcluster)  [unwired: 6 in, 2 out]
              }
            }
            n120 = for {
              N: 4 -> [_]
              tunnel: w289 -> [w329] mode=indexing
              tunnel: w279 -> [w330] mode=indexing
              tunnel: w281 -> [w328] mode=indexing
              tunnel: [w327] -> w287 mode=indexing
              n121 = case shown="True" w330 {
                tunnel: w329 -> [w331 w334]
                tunnel: w328 -> [_ w333]
                tunnel: [w331 w332] -> w327
                frame False {
                }
                frame True {
                  n122 = Bundle By Name(cluster=w334, "Pressure and Leak Test"=w333) -> (w332:T6)
                }
              }
            }
            n123 = Select(t=Process_Turbo."Rinse Wells" ("State In 2"), s=w294, f=Process_Turbo."Prime System" ("State In 2")) -> (s? t:f=w293:T1)
            n124 = Select(t=w293, s=w283, f=Process_Turbo."Idle" ("State In 2")) -> (s? t:f=w277:T1)
            n125 = Select(t=w277, s=w278, f=Process_Turbo."Idle" ("State In 2")) -> (s? t:f=w276:T1)
            n126 = Select(t=Process_Turbo."Error" ("State In 2"), s=w274, f=w276) -> (s? t:f=w295:T1)
          }
          frame "Prime System" {
            n127 = call "DAQ Manager.vi"("DAQ Mngr Action"=DAQ_Mngr."Pinch Valve Engage", "error in (no error)"=w337) -> ("error out"=w336:errorcluster)  [unwired: 6 in, 7 out]
            n128 = call "Update Cart Status.vi"("Selection"=status_update."Main Status", "error in (no error)"=w336, "String"="Clearing wells and lines" ("Reagent"), "FP"=w348) -> ("error out"=w341:errorcluster)  [unwired: 7 in]
            n129 = call "Run Script.vi"("Script Name"="Drain All Wells" ("name or relative path"), "Main References"=w348, "error in (no error)"=w341) -> ("error out"=w352:errorcluster)  [unwired: 8 in]
            n130 = call "Update Cart Status.vi"("Selection"=status_update."Main Status", "error in (no error)"=w352, "String"="Priming input lines" ("Reagent"), "FP"=w348) -> ("error out"=w350:errorcluster)  [unwired: 7 in]
            n131 = call "Run Script.vi"("Script Name"="Prime Input Lines" ("name or relative path"), "Main References"=w348, "error in (no error)"=w350) -> ("error out"=w345:errorcluster)  [unwired: 8 in]
            n132 = for {
              tunnel: w354 -> [w377] mode=indexing
              tunnel: [w376] -> w353 mode=indexing
              n133 = Bundle By Name(cluster=w377, "Primed"=TRUE) -> (w376:T6)
            }
            n134 = flat-sequence {
              tunnel: w347 -> [w374]
              tunnel: [w367] -> w346
              tunnel: w345 -> [w366]
              tunnel: [w365] -> w344
              frame #0 {
                n135 = Tick Count (ms)() -> (millisecond timer value=w365:u32)
                n136 = Subtract(x=w365, y=w374) -> (x-y=w362:u32)
                n137 = Divide(x=w362, y=u32 1000) -> (x/y=w364:dbl)
                n138 = call "Time Left Calc.vi"("Enum"=Time_elapsed."Update", "error in (no error)"=w366, "Time"=w364) -> ("error out"=w373:errorcluster)  [unwired: 6 in, 2 out]
                n139 = call "Time Left Calc.vi"("Enum"=Time_elapsed."Read", "error in (no error)"=w373) -> ("error out"=w371:errorcluster, "Time Left"=w372:u32)  [unwired: 7 in, 1 out]
                n140 = call "Time Left Calc.vi"("Enum"=Time_elapsed."Start", "error in (no error)"=w371, "Time"=w372) -> ("error out"=w367:errorcluster)  [unwired: 6 in, 2 out]
              }
            }
            n141 = Select(t=Process_Turbo."Rinse Wells" ("State In 2"), s=w360, f=Process_Turbo."Idle" ("State In 2")) -> (s? t:f=w361:T1)
          }
          frame "Rinse Wells" {
            n142 = call "Update Cart Status.vi"("Selection"=status_update."Main Status", "error in (no error)"=w400, "String"="Draining Wells" ("Reagent"), "FP"=w384) -> ("error out"=w399:errorcluster)  [unwired: 7 in]
            n143 = call "Run Script.vi"("Script Name"="Drain All Wells" ("name or relative path"), "Main References"=w384, "error in (no error)"=w399) -> ("error out"=w385:errorcluster)  [unwired: 8 in]
            n144 = call "Update Cart Status.vi"("Selection"=status_update."Main Status", "error in (no error)"=w385, "String"="Rinsing Syringe" ("Reagent"), "FP"=w384) -> ("error out"=w392:errorcluster)  [unwired: 7 in]
            n145 = for {
              N: 3 -> [_]
              tunnel: "Rinse Syringe" ("name or relative path") -> [w424]
              shift-right: [w423] -> w389
              shift-left: w392 -> [w425]
              tunnel: w384 -> [w422]
              n146 = call "Run Script.vi"("Script Name"=w424, "Main References"=w422, "error in (no error)"=w425) -> ("error out"=w423:errorcluster)  [unwired: 8 in]
            }
            n147 = call "Update Cart Status.vi"("Selection"=status_update."Main Status", "error in (no error)"=w389, "String"="Rinsing all wells" ("Reagent"), "FP"=w384) -> ("error out"=w394:errorcluster)  [unwired: 7 in]
            n148 = for {
              N: 4 -> [_]
              shift-right: [w426] -> w381
              shift-left: w394 -> [w429]
              tunnel: w384 -> [w427]
              tunnel: "Rinse All Wells" ("Script Name") -> [w428]
              n149 = call "Run Script.vi"("Script Name"=w428, "Main References"=w427, "error in (no error)"=w429) -> ("error out"=w426:errorcluster)  [unwired: 8 in]
            }
            n150 = flat-sequence {
              tunnel: w383 -> [w421]
              tunnel: [w414] -> w382
              tunnel: w381 -> [w413]
              tunnel: [w412] -> w380
              frame #0 {
                n151 = Tick Count (ms)() -> (millisecond timer value=w412:u32)
                n152 = Subtract(x=w412, y=w421) -> (x-y=w409:u32)
                n153 = Divide(x=w409, y=u32 1000) -> (x/y=w411:dbl)
                n154 = call "Time Left Calc.vi"("Enum"=Time_elapsed."Update", "error in (no error)"=w413, "Time"=w411) -> ("error out"=w416:errorcluster)  [unwired: 6 in, 2 out]
                n155 = call "Time Left Calc.vi"("Enum"=Time_elapsed."Read", "error in (no error)"=w416) -> ("error out"=w419:errorcluster, "Time Left"=w418:u32)  [unwired: 7 in, 1 out]
                n156 = call "Time Left Calc.vi"("Enum"=Time_elapsed."Start", "error in (no error)"=w419, "Time"=w418) -> ("error out"=w414:errorcluster)  [unwired: 6 in, 2 out]
              }
            }
            n157 = Select(t=Process_Turbo."Fill Wells" ("State In 2"), s=w406, f=Process_Turbo."Idle" ("State In 2")) -> (s? t:f=w408:T1)
          }
          frame "PrePresTest" {
            n158 = Unbundle By Name(w449) -> ("Config"=w456:refnum<vi>)
            n159 = property class="Clust (strict)"(reference=w456) -> ("Value"=w455:T2)  [unwired: 1 in, 2 out]
            n160 = Unbundle By Name(w455) -> ("TW Position"=w450:dbl, "Load Position"=w443:dbl)
            n161 = call "Update Cart Status.vi"("Selection"=status_update."Main Status", "error in (no error)"=w458, "String"="Testing for leaks and clogs", "FP"=w449) -> ("error out"=w451:errorcluster)  [unwired: 7 in]
            n162 = call "Detect Transition to TW.vi"("Main References"=w449, "error in (no error)"=w451, "Cart Array"=w446) -> ("error out"=w441:errorcluster, "Analysis"=w444:T7[])  [unwired: 7 in]
            n163 = case shown="True" TRUE {
              tunnel: w444 -> [_ w489]
              tunnel: w444 -> [_ w488]
              tunnel: w446 -> [w484 w487]
              tunnel: w449 -> [_ w486]
              tunnel: [w484 w485] -> w436
              frame False {
              }
              frame True {
                n164 = for {
                  tunnel: w489 -> [w495] mode=indexing
                  tunnel: w488 -> [w493] mode=indexing
                  tunnel: w487 -> [w494] mode=indexing
                  tunnel: w486 -> [w492]
                  tunnel: [w490] -> w485 mode=indexing
                  i -> [w491]
                  n165 = case shown="True" w494 {
                    selector: w494 -> [w496 _]
                    tunnel: w495 -> [_ w512]
                    tunnel: w493 -> [_ w511]
                    tunnel: w492 -> [_ w508]
                    tunnel: w491 -> [_ w507]
                    tunnel: [w496 w505] -> w490
                    frame False {
                    }
                    frame True {
                      n166 = Unbundle By Name(w512) -> ("Pressure"=w510:bool)
                      n167 = Unbundle By Name(w511) -> ("Decay"=w498:bool, "Pressure"=w509:bool)
                      n168 = Increment(x=w507) -> (x+1=w504:i32)
                      n169 = And(x=w510, y=w509) -> (x .and. y?=w499:bool)
                      n170 = Select(t="Test Passed" ("String"), s=w498, f="Clog Detected" ("String")) -> (s? t:f=w501:string)
                      n171 = And(x=w499, y=w498) -> (x .and. y?=w497:bool)
                      n172 = Select(t=w501, s=w499, f="Pressure Level Fail" ("String")) -> (s? t:f=w506:string)
                      n173 = case shown="False" w497 {
                        selector: w497 -> [w514 w518]
                        tunnel: w508 -> [w517 _]
                        tunnel: w504 -> [w516 _]
                        tunnel: w506 -> [w515 _]
                        tunnel: [w514 w518] -> w505
                        frame False {
                          n174 = call "Update 1 Cart Status.vi"("Selection"=Update_Single_Cart."Cart Status", "FP"=w517, "String"=w515, "Cartridge"=w516) -> ()  [unwired: 7 in, 1 out]
                        }
                        frame True {
                        }
                      }
                    }
                  }
                }
              }
            }
            n175 = flat-sequence {
              tunnel: [w469] -> w440
              tunnel: [w468] -> w439
              tunnel: w441 -> [w464]
              tunnel: w438 -> [w463]
              frame #0 {
                n176 = Tick Count (ms)() -> (millisecond timer value=w468:u32)
                n177 = Subtract(x=w468, y=w463) -> (x-y=w465:u32)
                n178 = Divide(x=w465, y=u32 1000) -> (x/y=w467:dbl)
                n179 = call "Time Left Calc.vi"("Enum"=Time_elapsed."Update", "error in (no error)"=w464, "Time"=w467) -> ("error out"=w471:errorcluster)  [unwired: 6 in, 2 out]
                n180 = call "Time Left Calc.vi"("Enum"=Time_elapsed."Read", "error in (no error)"=w471) -> ("error out"=w474:errorcluster, "Time Left"=w473:u32)  [unwired: 7 in, 1 out]
                n181 = call "Time Left Calc.vi"("Enum"=Time_elapsed."Start", "error in (no error)"=w474, "Time"=w473) -> ("error out"=w469:errorcluster)  [unwired: 6 in, 2 out]
              }
            }
            n182 = case shown="True" w447 {
              tunnel: w450 -> [w478 _]
              tunnel: w440 -> [w477 w482]
              tunnel: [w476 w481] -> w442
              tunnel: w443 -> [_ w480]
              frame True {
                n183 = call "Zaber Manager.vi"("Action"=Mot_Stage_Mngr."Abs Move", "Value"=w478, "error in (no error)"=w477) -> ("error out"=w476:errorcluster)  [unwired: 6 in, 6 out]
              }
              frame False {
                n184 = call "Zaber Manager.vi"("Action"=Mot_Stage_Mngr."Abs Move", "Value"=w480, "error in (no error)"=w482) -> ("error out"=w481:errorcluster)  [unwired: 6 in, 6 out]
              }
            }
            n185 = for {
              N: 4 -> [_]
              tunnel: w453 -> [w523] mode=indexing
              tunnel: [w524] -> w452 mode=indexing
              tunnel: w454 -> [w519]
              tunnel: w444 -> [w520] mode=indexing
              n186 = Unbundle By Name(w523) -> ("Test Array Pre"=w522:T7[])
              n187 = Insert Into Array(array=w522, index=w519, new element=w520) -> (w521:T7[])
              n188 = Bundle By Name(cluster=w523, "Test Array Pre"=w521) -> (w524:T6)
            }
            n189 = Select(t=Process_Turbo."Fill Wells" ("State In 2"), s=w447, f=Process_Turbo."Idle" ("State In 2")) -> (s? t:f=w435:T1)
            n190 = Or Array Elements(Boolean array=w436) -> (logical OR=w437:bool)
            n191 = Select(t=w435, s=w437, f=Process_Turbo."Abort" ("State In 2")) -> (s? t:f=w434:T1)
            n192 = Select(t=Process_Turbo."Error" ("State In 2"), s=w442, f=w434) -> (s? t:f=w461:T1)
          }
          frame "Fill Wells" {
            # "Move to TW position if we are not doing liquid check"
            n193 = Index Array(array=w541, index=w545) -> (element=w544:T10)
            n194 = Unbundle By Name(w544) -> ("Reagent"=w535:string, "Bottle"=w543:T30)
            n195 = call "Update Cart Status.vi"("Selection"=status_update."Reagent", "error in (no error)"=w536, "String"=w535, "Array"=w534, "FP"=w532) -> ("error out"=w533:errorcluster)  [unwired: 6 in]
            n196 = case shown="\"Bottle 4\"" w543 {
              tunnel: [Bottles."Bottle 1" ("Bottle X") Bottles."Bottle 2" ("Bottle X") Bottles."Bottle 3" ("Bottle X") Bottles."H2O" ("Bottle X")] -> w538
              frame "Bottle 1" {
              }
              frame "Bottle 2" {
              }
              frame "Bottle 3" {
              }
              frame "Bottle 4" {
              }
            }
            n197 = for {
              N: 4 -> [_]
              tunnel: w534 -> [w577] mode=indexing
              tunnel: w538 -> [w578]
              shift-right: [w579] -> w542
              shift-left: w533 -> [w575]
              tunnel: w532 -> [w574]
              tunnel: w535 -> [w573]
              i -> [w576]
              n198 = case shown="True" w577 {
                tunnel: w575 -> [w580 w589]
                tunnel: w576 -> [_ w581]
                tunnel: [w580 w592] -> w579
                tunnel: w578 -> [_ w590]
                tunnel: w574 -> [_ w586]
                tunnel: w573 -> [_ w584]
                frame False {
                }
                frame True {
                  n199 = Increment(x=w581) -> (x+1=w583:i32)
                  n200 = Format Into String(format string="Filling well %d with %s", w583, w584) -> (resulting string=w582:string)  [unwired: 2 in, 1 out]
                  n201 = call "Update Cart Status.vi"("Selection"=status_update."Main Status", "error in (no error)"=w589, "String"=w582, "FP"=w586) -> ("error out"=w588:errorcluster)  [unwired: 7 in]
                  n202 = call "Run Script.vi"("Script Name"="Fill Well_X Reagent_X" ("name or relative path"), "Main References"=w586, "error in (no error)"=w588, "Drain X"=w581, "Well X"=w581, "Bottle X"=w590) -> ("error out"=w592:errorcluster)  [unwired: 5 in]
                }
              }
            }
            n203 = case shown="True" FALSE {
              tunnel: w542 -> [w564 w567]
              tunnel: [w564 w566] -> w529
              tunnel: w532 -> [_ w565]
              frame False {
              }
              frame True {
                n204 = call "Run Script.vi"("Script Name"="Move to TW" ("name or relative path"), "Main References"=w565, "error in (no error)"=w567) -> ("error out"=w566:errorcluster)  [unwired: 8 in]
              }
            }
            n205 = flat-sequence {
              tunnel: [w557] -> w531
              tunnel: [w556] -> w530
              tunnel: w529 -> [w552]
              tunnel: w528 -> [w551]
              frame #0 {
                n206 = Tick Count (ms)() -> (millisecond timer value=w556:u32)
                n207 = Subtract(x=w556, y=w551) -> (x-y=w553:u32)
                n208 = Divide(x=w553, y=u32 1000) -> (x/y=w555:dbl)
                n209 = call "Time Left Calc.vi"("Enum"=Time_elapsed."Update", "error in (no error)"=w552, "Time"=w555) -> ("error out"=w559:errorcluster)  [unwired: 6 in, 2 out]
                n210 = call "Time Left Calc.vi"("Enum"=Time_elapsed."Read", "error in (no error)"=w559) -> ("error out"=w562:errorcluster, "Time Left"=w561:u32)  [unwired: 7 in, 1 out]
                n211 = call "Time Left Calc.vi"("Enum"=Time_elapsed."Start", "error in (no error)"=w562, "Time"=w561) -> ("error out"=w557:errorcluster)  [unwired: 6 in, 2 out]
              }
            }
            n212 = Select(t=Process_Turbo."High Vac On" ("State In 2"), s=w548, f=Process_Turbo."Idle" ("State In 2")) -> (s? t:f=w547:T1)
            n213 = Select(t=Process_Turbo."Error" ("State In 2"), s=w529, f=w547) -> (s? t:f=w546:T1)
          }
          frame "High Vac On" {
            n214 = call "Update Cart Status.vi"("Selection"=status_update."Main Status", "error in (no error)"=w617, "String"="Cleaning loading cap" ("Reagent"), "FP"=w606) -> ("error out"=w600:errorcluster)  [unwired: 7 in]
            n215 = Unbundle By Name(w606) -> ("Config"=w605:refnum<vi>)
            n216 = property class="Clust (strict)"(reference=w605) -> ("Value"=w604:T2)  [unwired: 1 in, 2 out]
            n217 = Unbundle By Name(w604) -> ("Load Position"=w601:dbl)
            n218 = Index Array(array=w621, index=w626) -> (element=w627:T10)
            n219 = call "DAQ Manager.vi"("DAQ Mngr Action"=DAQ_Mngr."Pinch Valve Disengage", "error in (no error)"=w600) -> ("error out"=w599:errorcluster)  [unwired: 6 in, 7 out]
            n220 = Unbundle By Name(w627) -> ("Wash Time(s)"=→"Wash Time(s)":dbl)
            n221 = call "Zaber Manager.vi"("Action"=Mot_Stage_Mngr."Abs Move", "Value"=w601, "error in (no error)"=w599) -> ("error out"=w602:errorcluster)  [unwired: 6 in, 6 out]
            n222 = call "16CH Denkovi Manager.vi"("Action"=16CH_Denkovi_Mngr."Vac ON", "error in (no error)"=w602, "Relays In"=w614) -> ("error out"=w625:errorcluster)  [unwired: 6 in, 2 out]
            n223 = flat-sequence {
              tunnel: w625 -> [w634]
              tunnel: [w634] -> w624
              tunnel: [w633] -> w623
              frame #0 {
                n224 = Tick Count (ms)() -> (millisecond timer value=w633:u32)
              }
            }
            n225 = while {
              tunnel: w624 -> [w652]
              tunnel: [w646] -> w596
              tunnel: w623 -> [w656]
              tunnel: w622 -> [_]
              tunnel: w606 -> [w645]
              tunnel: w614 -> [w644]
              tunnel: [w637] -> w607
              stop <- w653 stop-if-true
              n226 = call "DAQ Manager.vi"("DAQ Mngr Action"=DAQ_Mngr."Analyze Pres&Vac", "error in (no error)"=w652) -> ("error out"=w651:errorcluster)  [unwired: 6 in, 7 out]
              n227 = flat-sequence {
                tunnel: w651 -> [w658]
                tunnel: [w658] -> w647
                tunnel: [w657] -> w637
                frame #0 {
                  n228 = Tick Count (ms)() -> (millisecond timer value=w657:u32)
                }
              }
              n229 = expression code="x*1000"(20.0 ("Wash Time(s)")) -> (w643:dbl)
              n230 = Subtract(x=w637, y=w656) -> (x-y=w639:u32)
              n231 = Subtract(x=w643, y=w639) -> (x-y=w642:dbl)
              n232 = expression code="x/1000"(w639) -> (w638:u32)
              n233 = expression code="x/1000"(w642) -> (w641:dbl)
              n234 = global read "Main Globals.vi" "Cancel"() -> (w655:bool)
              n235 = call "Time Left Calc.vi"("Enum"=Time_elapsed."Update", "Time"=w638) -> ()  [unwired: 7 in, 3 out]
              n236 = Format Into String(format string="%.1f seconds", w641) -> (resulting string=w648:string)  [unwired: 2 in, 1 out]
              n237 = Greater?(x=w639, y=w643) -> (0:w654:bool)
              n238 = Compound Arithmetic op=OR(w654, w655) -> (w653:bool)
              n239 = call "Update Cart Status.vi"("Selection"=status_update."Cartridge", "error in (no error)"=w647, "String"=w648, "Array"=w644, "FP"=w645) -> ("error out"=w646:errorcluster)  [unwired: 6 in]
            }
            n240 = call "Update Cart Status.vi"("Selection"=status_update."Cartridge", "error in (no error)"=w596, "String"="TW in progress", "Array"=w614, "FP"=w606) -> ("error out"=w613:errorcluster)  [unwired: 6 in]
            n241 = call "Time Left Calc.vi"("Enum"=Time_elapsed."Read", "error in (no error)"=w613) -> ("error out"=w611:errorcluster, "Time Left"=w609:u32)  [unwired: 7 in, 1 out]
            n242 = call "Time Left Calc.vi"("Enum"=Time_elapsed."Start", "error in (no error)"=w611, "Time"=w609) -> ("error out"=w608:errorcluster)  [unwired: 6 in, 2 out]
            n243 = Select(t=Process_Turbo."Pressure&Vac Load" ("State In 2"), s=w631, f=Process_Turbo."Idle" ("State In 2")) -> (s? t:f=w630:T1)
            n244 = Select(t=Process_Turbo."Error" ("State In 2"), s=w608, f=w630) -> (s? t:f=w629:T1)
          }
          frame "Pressure&Vac Load" {
            n245 = call "Update Cart Status.vi"("Selection"=status_update."Main Status", "error in (no error)"=w685, "String"="Applying pressure and vac" ("Reagent"), "FP"=w675) -> ("error out"=w669:errorcluster)  [unwired: 7 in]
            n246 = Unbundle By Name(w675) -> ("Config"=w674:refnum<vi>)
            n247 = property class="Clust (strict)"(reference=w674) -> ("Value"=w673:T2)  [unwired: 1 in, 2 out]
            n248 = Unbundle By Name(w673) -> ("TW Position"=w670:dbl)
            n249 = call "DAQ Manager.vi"("DAQ Mngr Action"=DAQ_Mngr."Pinch Valve Engage", "error in (no error)"=w669) -> ("error out"=w668:errorcluster)  [unwired: 6 in, 7 out]
            n250 = Index Array(array=w689, index=w694) -> (element=w695:T10)
            n251 = Unbundle By Name(w695) -> ("Wash Time(s)"=→"Wash Time(s) 2":dbl)
            n252 = call "Zaber Manager.vi"("Action"=Mot_Stage_Mngr."Abs Move", "Value"=w670, "error in (no error)"=w668) -> ("error out"=w671:errorcluster)  [unwired: 6 in, 6 out]
            n253 = call "16CH Denkovi Manager.vi"("Action"=16CH_Denkovi_Mngr."Pres ON", "error in (no error)"=w671, "Relays In"=w662) -> ("error out"=w693:errorcluster)  [unwired: 6 in, 2 out]
            n254 = flat-sequence {
              tunnel: w693 -> [w702]
              tunnel: [w702] -> w692
              tunnel: [w701] -> w691
              frame #0 {
                n255 = Tick Count (ms)() -> (millisecond timer value=w701:u32)
              }
            }
            n256 = while {
              tunnel: w692 -> [w720]
              tunnel: [w714] -> w665
              tunnel: w691 -> [w724]
              tunnel: w690 -> [_]
              tunnel: w675 -> [w713]
              tunnel: w662 -> [w712]
              tunnel: [w705] -> w676
              stop <- w721 stop-if-true
              n257 = call "DAQ Manager.vi"("DAQ Mngr Action"=DAQ_Mngr."Analyze Pres&Vac", "error in (no error)"=w720) -> ("error out"=w719:errorcluster)  [unwired: 6 in, 7 out]
              n258 = flat-sequence {
                tunnel: w719 -> [w726]
                tunnel: [w726] -> w715
                tunnel: [w725] -> w705
                frame #0 {
                  n259 = Tick Count (ms)() -> (millisecond timer value=w725:u32)
                }
              }
              n260 = expression code="x*1000"(20.0 ("Wash Time(s)")) -> (w711:dbl)
              n261 = Subtract(x=w705, y=w724) -> (x-y=w707:u32)
              n262 = Subtract(x=w711, y=w707) -> (x-y=w710:dbl)
              n263 = expression code="x/1000"(w707) -> (w706:u32)
              n264 = expression code="x/1000"(w710) -> (w709:dbl)
              n265 = global read "Main Globals.vi" "Cancel"() -> (w723:bool)
              n266 = call "Time Left Calc.vi"("Enum"=Time_elapsed."Update", "Time"=w706) -> ()  [unwired: 7 in, 3 out]
              n267 = Format Into String(format string="%.1f seconds", w709) -> (resulting string=w716:string)  [unwired: 2 in, 1 out]
              n268 = Greater?(x=w707, y=w711) -> (0:w722:bool)
              n269 = Compound Arithmetic op=OR(w722, w723) -> (w721:bool)
              n270 = call "Update Cart Status.vi"("Selection"=status_update."Cartridge", "error in (no error)"=w715, "String"=w716, "Array"=w712, "FP"=w713) -> ("error out"=w714:errorcluster)  [unwired: 6 in]
            }
            n271 = call "16CH Denkovi Manager.vi"("Action"=16CH_Denkovi_Mngr."Pres Vent&Close", "error in (no error)"=w665, "Relays In"=w662) -> ("error out"=w664:errorcluster)  [unwired: 6 in, 2 out]
            n272 = call "Update Cart Status.vi"("Selection"=status_update."Cartridge", "error in (no error)"=w664, "String"="TW in progress", "Array"=w662, "FP"=w675) -> ("error out"=w682:errorcluster)  [unwired: 6 in]
            n273 = call "Time Left Calc.vi"("Enum"=Time_elapsed."Read", "error in (no error)"=w682) -> ("error out"=w680:errorcluster, "Time Left"=w678:u32)  [unwired: 7 in, 1 out]
            n274 = call "Time Left Calc.vi"("Enum"=Time_elapsed."Start", "error in (no error)"=w680, "Time"=w678) -> ("error out"=w677:errorcluster)  [unwired: 6 in, 2 out]
            n275 = Select(t=Process_Turbo."Trap Vac" ("State In 2"), s=w699, f=Process_Turbo."Idle" ("State In 2")) -> (s? t:f=w698:T1)
            n276 = Select(t=Process_Turbo."Error" ("State In 2"), s=w677, f=w698) -> (s? t:f=w697:T1)
          }
          frame "Trap Vac" {
            n277 = call "Update Cart Status.vi"("Selection"=status_update."Main Status", "error in (no error)"=w753, "String"="Trapping vacuum" ("Reagent"), "FP"=w742) -> ("error out"=w737:errorcluster)  [unwired: 7 in]
            n278 = Unbundle By Name(w742) -> ("Config"=w741:refnum<vi>)
            n279 = property class="Clust (strict)"(reference=w741) -> ("Value"=w740:T2)  [unwired: 1 in, 2 out]
            n280 = Unbundle By Name(w740) -> ("Load Position"=w738:dbl)
            n281 = Index Array(array=w758, index=w763) -> (element=w764:T10)
            n282 = call "DAQ Manager.vi"("DAQ Mngr Action"=DAQ_Mngr."Pinch Valve Disengage", "error in (no error)"=w737) -> ("error out"=w735:errorcluster)  [unwired: 6 in, 7 out]
            n283 = Unbundle By Name(w764) -> ("Wash Time(s)"=w759:dbl)
            n284 = call "Delay with Error Handling.vi"("error in (no error)"=w735, "Delay (ms)"=u32 3000) -> ("error out"=w734:errorcluster)  [unwired: 9 in]
            n285 = call "Zaber Manager.vi"("Action"=Mot_Stage_Mngr."Abs Move", "Value"=w738, "error in (no error)"=w734) -> ("error out"=w732:errorcluster)  [unwired: 6 in, 6 out]
            n286 = call "16CH Denkovi Manager.vi"("Action"=16CH_Denkovi_Mngr."Vac Vent&Close", "error in (no error)"=w732) -> ("error out"=w731:errorcluster)  [unwired: 7 in, 2 out]
            n287 = flat-sequence {
              tunnel: w731 -> [w770]
              tunnel: [w770] -> w762
              tunnel: [w769] -> w761
              frame #0 {
                n288 = Tick Count (ms)() -> (millisecond timer value=w769:u32)
              }
            }
            n289 = while {
              tunnel: w762 -> [w787]
              tunnel: [w781] -> w730
              tunnel: w761 -> [w792]
              tunnel: w760 -> [_]
              tunnel: w759 -> [w791]
              tunnel: w742 -> [w780]
              tunnel: w750 -> [w779]
              tunnel: [w772] -> w743
              stop <- w788 stop-if-true
              n290 = call "DAQ Manager.vi"("DAQ Mngr Action"=DAQ_Mngr."Analyze Pres&Vac", "error in (no error)"=w787) -> ("error out"=w786:errorcluster)  [unwired: 6 in, 7 out]
              n291 = flat-sequence {
                tunnel: w786 -> [w794]
                tunnel: [w794] -> w782
                tunnel: [w793] -> w772
                frame #0 {
                  n292 = Tick Count (ms)() -> (millisecond timer value=w793:u32)
                }
              }
              n293 = expression code="x*1000"(w791) -> (w778:dbl)
              n294 = Subtract(x=w772, y=w792) -> (x-y=w774:u32)
              n295 = Subtract(x=w778, y=w774) -> (x-y=w777:dbl)
              n296 = expression code="x/1000"(w774) -> (w773:u32)
              n297 = expression code="x/1000"(w777) -> (w776:dbl)
              n298 = global read "Main Globals.vi" "Cancel"() -> (w790:bool)
              n299 = call "Time Left Calc.vi"("Enum"=Time_elapsed."Update", "Time"=w773) -> ()  [unwired: 7 in, 3 out]
              n300 = Format Into String(format string="%.1f seconds", w776) -> (resulting string=w783:string)  [unwired: 2 in, 1 out]
              n301 = Greater?(x=w774, y=w778) -> (0:w789:bool)
              n302 = Compound Arithmetic op=OR(w789, w790) -> (w788:bool)
              n303 = call "Update Cart Status.vi"("Selection"=status_update."Cartridge", "error in (no error)"=w782, "String"=w783, "Array"=w779, "FP"=w780) -> ("error out"=w781:errorcluster)  [unwired: 6 in]
            }
            n304 = call "Update Cart Status.vi"("Selection"=status_update."Cartridge", "error in (no error)"=w730, "String"="TW in progress", "Array"=w750, "FP"=w742) -> ("error out"=w749:errorcluster)  [unwired: 6 in]
            n305 = call "Time Left Calc.vi"("Enum"=Time_elapsed."Read", "error in (no error)"=w749) -> ("error out"=w747:errorcluster, "Time Left"=w745:u32)  [unwired: 7 in, 1 out]
            n306 = call "Time Left Calc.vi"("Enum"=Time_elapsed."Start", "error in (no error)"=w747, "Time"=w745) -> ("error out"=w744:errorcluster)  [unwired: 6 in, 2 out]
            n307 = Select(t=Process_Turbo."Drain&Rinse" ("State In 2"), s=w767, f=Process_Turbo."Idle" ("State In 2")) -> (s? t:f=w766:T1)
            n308 = Select(t=Process_Turbo."Error" ("State In 2"), s=w744, f=w766) -> (s? t:f=w765:T1)
          }
          frame "PostPresTest" {
            n309 = Unbundle By Name(w812) -> ("Config"=w818:refnum<vi>)
            n310 = property class="Clust (strict)"(reference=w818) -> ("Value"=w817:T2)  [unwired: 1 in, 2 out]
            n311 = Unbundle By Name(w817) -> ("Load Position"=w813:dbl)
            n312 = call "Update Cart Status.vi"("Selection"=status_update."Main Status", "error in (no error)"=w820, "String"="Testing for leaks and clogs", "FP"=w812) -> ("error out"=w806:errorcluster)  [unwired: 7 in]
            n313 = call "Detect Transition to Load.vi"("Main References"=w812, "error in (no error)"=w806, "Cart Array"=w798) -> ("error out"=w804:errorcluster, "Analysis"=w805:T7[])  [unwired: 7 in]
            n314 = case shown="True" FALSE {
              tunnel: w805 -> [_ w849]
              tunnel: w805 -> [_ w848]
              tunnel: w798 -> [w844 w847]
              tunnel: w812 -> [_ w846]
              tunnel: [w844 w845] -> w811
              frame False {
              }
              frame True {
                n315 = for {
                  tunnel: w849 -> [w855] mode=indexing
                  tunnel: w848 -> [w853] mode=indexing
                  tunnel: w847 -> [w854] mode=indexing
                  tunnel: w846 -> [w852]
                  tunnel: [w850] -> w845 mode=indexing
                  i -> [w851]
                  n316 = case shown="True" w854 {
                    selector: w854 -> [w856 _]
                    tunnel: w855 -> [_ w874]
                    tunnel: w853 -> [_ w873]
                    tunnel: w852 -> [_ w868]
                    tunnel: w851 -> [_ w866]
                    tunnel: [w856 w862] -> w850
                    frame False {
                    }
                    frame True {
                      n317 = Unbundle By Name(w874) -> ("Transition"=w872:bool, "Pressure"=w870:bool)
                      n318 = Unbundle By Name(w873) -> ("Transition"=w871:bool, "Pressure"=w869:bool)
                      n319 = Increment(x=w866) -> (x+1=w861:i32)
                      n320 = And(x=w870, y=w869) -> (x .and. y?=w865:bool)
                      n321 = And(x=w872, y=w871) -> (x .and. y?=w864:bool)
                      n322 = Select(t="Test Passed" ("String"), s=w864, f="Clog Detected" ("String")) -> (s? t:f=w858:string)
                      n323 = And(x=w864, y=w865) -> (x .and. y?=w867:bool)
                      n324 = Select(t=w858, s=w865, f="Pressure Level Fail" ("String")) -> (s? t:f=w863:string)
                      n325 = case shown="False" w867 {
                        selector: w867 -> [w876 w880]
                        tunnel: w868 -> [w879 _]
                        tunnel: w861 -> [w878 _]
                        tunnel: w863 -> [w877 _]
                        tunnel: [w876 w880] -> w862
                        frame False {
                          n326 = call "Update 1 Cart Status.vi"("Selection"=Update_Single_Cart."Cart Status", "FP"=w879, "String"=w877, "Cartridge"=w878) -> ()  [unwired: 7 in, 1 out]
                        }
                        frame True {
                        }
                      }
                    }
                  }
                }
              }
            }
            n327 = call "16CH Denkovi Manager.vi"("Action"=16CH_Denkovi_Mngr."Pres Vent&Close", "error in (no error)"=w804, "Relays In"=w798) -> ("error out"=w802:errorcluster)  [unwired: 6 in, 2 out]
            n328 = flat-sequence {
              tunnel: [w832] -> w801
              tunnel: [w831] -> w800
              tunnel: w802 -> [w827]
              tunnel: w799 -> [w826]
              frame #0 {
                n329 = Tick Count (ms)() -> (millisecond timer value=w831:u32)
                n330 = Subtract(x=w831, y=w826) -> (x-y=w828:u32)
                n331 = Divide(x=w828, y=u32 1000) -> (x/y=w830:dbl)
                n332 = call "Time Left Calc.vi"("Enum"=Time_elapsed."Update", "error in (no error)"=w827, "Time"=w830) -> ("error out"=w834:errorcluster)  [unwired: 6 in, 2 out]
                n333 = call "Time Left Calc.vi"("Enum"=Time_elapsed."Read", "error in (no error)"=w834) -> ("error out"=w837:errorcluster, "Time Left"=w836:u32)  [unwired: 7 in, 1 out]
                n334 = call "Time Left Calc.vi"("Enum"=Time_elapsed."Start", "error in (no error)"=w837, "Time"=w836) -> ("error out"=w832:errorcluster)  [unwired: 6 in, 2 out]
              }
            }
            n335 = for {
              N: 4 -> [_]
              tunnel: w815 -> [w885] mode=indexing
              tunnel: [w886] -> w814 mode=indexing
              tunnel: w816 -> [w881]
              tunnel: w805 -> [w882] mode=indexing
              n336 = Unbundle By Name(w885) -> ("Test Array Post"=w884:T7[])
              n337 = Insert Into Array(array=w884, index=w881, new element=w882) -> (w883:T7[])
              n338 = Bundle By Name(cluster=w885, "Test Array Post"=w883) -> (w886:T6)
            }
            n339 = case shown="True" w807 {
              tunnel: w813 -> [_ w842]
              tunnel: w801 -> [w839 w841]
              tunnel: [w839 w840] -> w809
              frame False {
              }
              frame True {
                n340 = call "Zaber Manager.vi"("Action"=Mot_Stage_Mngr."Abs Move", "Value"=w842, "error in (no error)"=w841) -> ("error out"=w840:errorcluster)  [unwired: 6 in, 6 out]
              }
            }
            n341 = Select(t=Process_Turbo."Drain&Rinse" ("State In 2"), s=w807, f=Process_Turbo."Idle" ("State In 2")) -> (s? t:f=w824:T1)
            n342 = Select(t=Process_Turbo."Error" ("State In 2"), s=w809, f=w824) -> (s? t:f=w823:T1)
          }
          frame "Drain&Rinse" {
            n343 = call "Update Cart Status.vi"("Selection"=status_update."Main Status", "error in (no error)"=w901, "String"="Draining Wells", "FP"=w902) -> ("error out"=w900:errorcluster)  [unwired: 7 in]
            n344 = Unbundle By Name(w902) -> ("Config"=w912:refnum<vi>)
            n345 = property class="Clust (strict)"(reference=w912) -> ("Value"=w911:T2)  [unwired: 1 in, 2 out]
            n346 = Unbundle By Name(w911) -> ("Load Position"=w910:dbl)
            n347 = Index Array(array=w918, index=w920) -> (element=w923:T10)
            n348 = call "Zaber Manager.vi"("Action"=Mot_Stage_Mngr."Abs Move", "Value"=w910, "error in (no error)"=w900) -> ("error out"=w906:errorcluster)  [unwired: 6 in, 6 out]
            n349 = Unbundle By Name(w923) -> ("# of Rinses"=w896:i16)
            n350 = for {
              N: 4 -> [_]
              shift-right: [w944] -> w905
              shift-left: w906 -> [w945]
              tunnel: w907 -> [w943] mode=indexing
              tunnel: w902 -> [w941]
              tunnel: "Drain Well X" ("Script Name") -> [w940]
              i -> [w942]
              n351 = case shown="True" w943 {
                tunnel: w945 -> [w946 w951]
                tunnel: [w946 w949] -> w944
                tunnel: w942 -> [_ w950]
                tunnel: w941 -> [_ w948]
                tunnel: w940 -> [_ w947]
                frame False {
                }
                frame True {
                  n352 = call "Run Script.vi"("Script Name"=w947, "Main References"=w948, "error in (no error)"=w951, "Drain X"=w950, "Well X"=w950) -> ("error out"=w949:errorcluster)  [unwired: 6 in]
                }
              }
            }
            n353 = case shown="False" w897 {
              tunnel: w896 -> [_ w939]
              tunnel: [i16 1 ("# of Rinses") w939] -> w895
              frame False {
              }
              frame True {
              }
            }
            n354 = case shown="Default" w895 {
              selector: w895 -> [_ w956]
              tunnel: w907 -> [_ w959]
              tunnel: w905 -> [w952 w953]
              tunnel: w902 -> [_ w958]
              tunnel: [w952 w957] -> w894
              tunnel: "Rinse Well X step1" ("Script Name") -> [_ w955]
              tunnel: "Rinse Well X step3" ("Script Name") -> [_ w954]
              frame 0 {
                # "skip rinsing if # of rinses is 0"
              }
              frame Default {
                n355 = for {
                  N: w956 -> [w968]
                  tunnel: w959 -> [w960]
                  tunnel: w958 -> [w961]
                  shift-right: [w970] -> w957
                  shift-left: w953 -> [w973]
                  tunnel: w955 -> [w964]
                  tunnel: w954 -> [w963]
                  i -> [w966]
                  n356 = Increment(x=w966) -> (x+1=w965:i32)
                  n357 = Format Into String(format string="Rinsing wells %d/%d", w965, w968) -> (resulting string=w967:string)  [unwired: 2 in, 1 out]
                  n358 = call "Update Cart Status.vi"("Selection"=status_update."Main Status", "error in (no error)"=w973, "String"=w967, "FP"=w961) -> ("error out"=w972:errorcluster)  [unwired: 7 in]
                  n359 = for {
                    N: 4 -> [_]
                    shift-right: [w992] -> w962
                    shift-left: w972 -> [w993]
                    tunnel: w960 -> [w991] mode=indexing
                    tunnel: w961 -> [w989]
                    tunnel: w964 -> [w988]
                    i -> [w990]
                    n360 = case shown="True" w991 {
                      tunnel: w993 -> [w994 w999]
                      tunnel: [w994 w997] -> w992
                      tunnel: w990 -> [_ w998]
                      tunnel: w989 -> [_ w996]
                      tunnel: w988 -> [_ w995]
                      frame False {
                      }
                      frame True {
                        n361 = call "Run Script.vi"("Script Name"=w995, "Main References"=w996, "error in (no error)"=w999, "Drain X"=w998, "Well X"=w998) -> ("error out"=w997:errorcluster)  [unwired: 6 in]
                      }
                    }
                  }
                  n362 = for {
                    N: 4 -> [_]
                    shift-right: [w980] -> w970
                    shift-left: w962 -> [w981]
                    tunnel: w960 -> [w979] mode=indexing
                    tunnel: w961 -> [w977]
                    tunnel: w963 -> [w976]
                    i -> [w978]
                    n363 = case shown="True" w979 {
                      tunnel: w981 -> [w982 w987]
                      tunnel: [w982 w985] -> w980
                      tunnel: w978 -> [_ w986]
                      tunnel: w977 -> [_ w984]
                      tunnel: w976 -> [_ w983]
                      frame False {
                      }
                      frame True {
                        n364 = call "Run Script.vi"("Script Name"=w983, "Main References"=w984, "error in (no error)"=w987, "Drain X"=w986, "Well X"=w986) -> ("error out"=w985:errorcluster)  [unwired: 6 in]
                      }
                    }
                  }
                }
              }
            }
            n365 = Increment(x=w920) -> (x+1=w919:i32)
            n366 = Array Size(array=w918) -> (size(s)=w921:i32)
            n367 = Greater?(x=w921, y=w919) -> (0:w917:bool)
            n368 = flat-sequence {
              tunnel: [w931] -> w893
              tunnel: [w930] -> w892
              tunnel: w894 -> [w926]
              tunnel: w891 -> [w925]
              frame #0 {
                n369 = Tick Count (ms)() -> (millisecond timer value=w930:u32)
                n370 = Subtract(x=w930, y=w925) -> (x-y=w927:u32)
                n371 = Divide(x=w927, y=u32 1000) -> (x/y=w929:dbl)
                n372 = call "Time Left Calc.vi"("Enum"=Time_elapsed."Update", "error in (no error)"=w926, "Time"=w929) -> ("error out"=w933:errorcluster)  [unwired: 6 in, 2 out]
                n373 = call "Time Left Calc.vi"("Enum"=Time_elapsed."Read", "error in (no error)"=w933) -> ("error out"=w936:errorcluster, "Time Left"=w935:u32)  [unwired: 7 in, 1 out]
                n374 = call "Time Left Calc.vi"("Enum"=Time_elapsed."Start", "error in (no error)"=w936, "Time"=w935) -> ("error out"=w931:errorcluster)  [unwired: 6 in, 2 out]
              }
            }
            n375 = Select(t=Process_Turbo."Fill Wells" ("State In 2"), s=w917, f=Process_Turbo."Dry" ("State In 2")) -> (s? t:f=w915:T1)
            n376 = Select(t=w915, s=w897, f=Process_Turbo."Idle" ("State In 2")) -> (s? t:f=w914:T1)
            n377 = Select(t=Process_Turbo."Error" ("State In 2"), s=w893, f=w914) -> (s? t:f=w922:T1)
          }
          frame "Dry" {
            n378 = Unbundle By Name(w1009) -> ("Config"=w1015:refnum<vi>)
            n379 = property class="Clust (strict)"(reference=w1015) -> ("Value"=w1013:T2)  [unwired: 1 in, 2 out]
            n380 = Unbundle By Name(w1013) -> ("Dry Time(s)"=w1012:dbl, "TW Position"=w1014:dbl)
            n381 = Format Into String(format string="Drying capillaries for %ds", w1012) -> (resulting string=w1010:string)  [unwired: 2 in, 1 out]
            n382 = call "Update Cart Status.vi"("Selection"=status_update."Main Status", "error in (no error)"=w1017, "String"=w1010, "FP"=w1009) -> ("error out"=w1016:errorcluster)  [unwired: 7 in]
            n383 = call "Zaber Manager.vi"("Action"=Mot_Stage_Mngr."Abs Move", "Value"=w1014, "error in (no error)"=w1016) -> ("error out"=w1023:errorcluster)  [unwired: 6 in, 6 out]
            n384 = call "16CH Denkovi Manager.vi"("Action"=16CH_Denkovi_Mngr."Pres ON", "error in (no error)"=w1023, "Relays In"=w1008) -> ("error out"=w1032:errorcluster)  [unwired: 6 in, 2 out]
            n385 = flat-sequence {
              tunnel: w1032 -> [w1036]
              tunnel: [w1036] -> w1031
              tunnel: [w1035] -> w1030
              frame #0 {
                n386 = Tick Count (ms)() -> (millisecond timer value=w1035:u32)
              }
            }
            n387 = while {
              tunnel: w1031 -> [w1053]
              tunnel: [w1050] -> w1028
              tunnel: w1030 -> [w1058]
              tunnel: w1008 -> [w1047]
              tunnel: w1029 -> [_]
              tunnel: w1012 -> [w1057]
              tunnel: w1009 -> [w1048]
              tunnel: [w1038] -> w1003
              stop <- w1054 stop-if-true
              n388 = call "DAQ Manager.vi"("DAQ Mngr Action"=DAQ_Mngr."Analyze Pres&Vac", "error in (no error)"=w1053) -> ("error out"=w1052:errorcluster)  [unwired: 6 in, 7 out]
              n389 = flat-sequence {
                tunnel: w1052 -> [w1060]
                tunnel: [w1060] -> w1051
                tunnel: [w1059] -> w1038
                frame #0 {
                  n390 = Tick Count (ms)() -> (millisecond timer value=w1059:u32)
                }
              }
              n391 = expression code="x*1000"(w1057) -> (w1042:dbl)
              n392 = Subtract(x=w1038, y=w1058) -> (x-y=w1041:u32)
              n393 = Subtract(x=w1042, y=w1041) -> (x-y=w1046:dbl)
              n394 = expression code="x/1000"(w1041) -> (w1040:u32)
              n395 = expression code="x/1000"(w1046) -> (w1045:dbl)
              n396 = Greater?(x=w1041, y=w1042) -> (0:w1055:bool)
              n397 = call "Time Left Calc.vi"("Enum"=Time_elapsed."Update", "Time"=w1040) -> ()  [unwired: 7 in, 3 out]
              n398 = Format Into String(format string="%.1f seconds", w1045) -> (resulting string=w1043:string)  [unwired: 2 in, 1 out]
              n399 = global read "Main Globals.vi" "Cancel"() -> (w1056:bool)
              n400 = call "Update Cart Status.vi"("Selection"=status_update."Cartridge", "error in (no error)"=w1051, "String"=w1043, "Array"=w1047, "FP"=w1048) -> ("error out"=w1050:errorcluster)  [unwired: 6 in]
              n401 = Compound Arithmetic op=OR(w1055, w1056) -> (w1054:bool)
            }
            n402 = call "16CH Denkovi Manager.vi"("Action"=16CH_Denkovi_Mngr."Pres Vent&Close", "error in (no error)"=w1028, "Relays In"=w1008) -> ("error out"=w1004:errorcluster)  [unwired: 6 in, 2 out]
            n403 = Select(t=Process_Turbo."Report" ("State In 2"), s=w1020, f=Process_Turbo."Idle" ("State In 2")) -> (s? t:f=w1026:T1)
            n404 = call "Time Left Calc.vi"("Enum"=Time_elapsed."Start", "error in (no error)"=w1004, "Time"=u32 0) -> ("error out"=w1005:errorcluster)  [unwired: 6 in, 2 out]
            n405 = Select(t=Process_Turbo."Error" ("State In 2"), s=w1005, f=w1026) -> (s? t:f=w1025:T1)
          }
          frame "Error" {
            # "TODO:  handle errors\nask user to remove cartridges"
            n406 = call "Data Logger.vi"("Action"=T16."Close", "error in"=w1065) -> ("error out"=w1064:errorcluster)  [unwired: 9 in]
            n407 = Unbundle By Name(w1067) -> ("Cartridges"=w1072:refnum<vi>)
            n408 = Unbundle By Name(w1067) -> ("Start TW"=w1074:refnum<vi>)
            n409 = property class="Bool (strict)"(reference=w1074, "Value"=FALSE) -> ()  [unwired: 1 in, 2 out]
            n410 = property class="Clust (strict)"(reference=w1072) -> (reference out=w1069:refnum<vi>, "Value"=w1071:T27)  [unwired: 1 in, 1 out]
            n411 = Bundle By Name(cluster=w1071, "Current Status"="Error has occured.  Process aborted") -> (w1068:T27)
            n412 = property class="Clust (strict)"(reference=w1069, "Value"=w1068) -> ()  [unwired: 1 in, 2 out]
          }
          frame "Abort" {
            n413 = call "Update Cart Status.vi"("Selection"=status_update."Main Status", "error in (no error)"=w1100, "String"="Aborting Run" ("Reagent"), "FP"=w1084) -> ("error out"=w1091:errorcluster)  [unwired: 7 in]
            n414 = Unbundle By Name(w1084) -> ("Start TW"=w1083:refnum<vi>)
            n415 = property class="Bool (strict)"(reference=w1083, "Value"=FALSE) -> ()  [unwired: 1 in, 2 out]
            n416 = call "Zaber Manager.vi"("Action"=Mot_Stage_Mngr."Home", "error in (no error)"=w1091) -> ("error out"=w1097:errorcluster)  [unwired: 7 in, 6 out]
            n417 = call "16CH Denkovi Manager.vi"("Action"=16CH_Denkovi_Mngr."Set Peristaltic", "error in (no error)"=w1097, "Relays In"=bool[] [FALSE, FALSE, FALSE, FALSE, FALSE, FALSE, FALSE, FALSE, FALSE, FALSE, FALSE, FALSE, FALSE, FALSE, FALSE, FALSE]) -> ("error out"=w1096:errorcluster)  [unwired: 6 in, 2 out]
            n418 = call "16CH Denkovi Manager.vi"("Action"=16CH_Denkovi_Mngr."Pres Vent&Close", "error in (no error)"=w1096, "Relays In"=bool[] [TRUE, TRUE, TRUE, TRUE, FALSE, FALSE, FALSE, FALSE, FALSE, FALSE, FALSE, FALSE, FALSE, FALSE, FALSE, FALSE]) -> ("error out"=w1095:errorcluster)  [unwired: 6 in, 2 out]
            n419 = call "Tecan Mngr.vi"("Mngr Action"=Tricon_Mngr."Start Pump", "Pump Data"=T23 {"Syringe Pos"=0, "Rate"=60.0, "Volume"=0.0, "Valve"=enum."Waste", "Action"=enum."Withdraw", "Move Type"=enum."Abs", "Init"=TRUE, "Empty Syr."=FALSE, "Full Fill"=FALSE, "Units"=enum."ul/s"}, "Pump Config"=w1090, "error in (no error)"=w1095) -> ("error out"=w1087:errorcluster)  [unwired: 6 in, 5 out]
            n420 = call "DAQ Manager.vi"("DAQ Mngr Action"=DAQ_Mngr."Pinch Valve Disengage", "error in (no error)"=w1087) -> ("error out"=w1086:errorcluster)  [unwired: 6 in, 7 out]
            n421 = call "Data Logger.vi"("Action"=T16."Close", "error in"=w1086) -> ("error out"=w1093:errorcluster)  [unwired: 9 in]
          }
          frame "Report" {
            n422 = Get Date/Time String(date format (0)=enum16{"short", "long", "abbreviated"}."short") -> (date string=w1125:string, time string=w1124:string)  [unwired: 2 in]
            n423 = Concatenate Strings(w1125, "   " ("string"), w1124) -> (w1122:string)
            n424 = for {
              tunnel: w1121 -> [w1153] mode=indexing
              tunnel: w1122 -> [w1152]
              tunnel: [w1151] -> w1119 mode=indexing
              tunnel: w1114 -> [w1150] mode=indexing
              n425 = case shown="True" w1150 {
                tunnel: w1153 -> [w1154 w1157]
                tunnel: w1152 -> [_ w1156]
                tunnel: [w1154 w1155] -> w1151
                frame False {
                }
                frame True {
                  n426 = Bundle By Name(cluster=w1157, "Finish Timestamp"=w1156) -> (w1155:T6)
                }
              }
            }
            n427 = call "Data Logger.vi"("Action"=T16."Close", "error in"=w1118) -> ("error out"=w1117:errorcluster)  [unwired: 9 in]
            n428 = for {
              N: 4 -> [_]
              tunnel: w1117 -> [w1136]
              tunnel: [w1135] -> w1120
              tunnel: w1114 -> [w1134] mode=indexing
              tunnel: w1119 -> [w1133] mode=indexing
              tunnel: w1116 -> [w1132]
              i -> [w1131]
              n429 = case shown="True" w1134 {
                tunnel: w1136 -> [w1137 w1149]
                tunnel: [w1137 w1146] -> w1135
                tunnel: w1133 -> [_ w1148]
                tunnel: w1132 -> [_ w1145]
                tunnel: w1131 -> [_ w1143]
                frame False {
                }
                frame True {
                  n430 = call "Create Summary File.vi"("FP"=w1145, "error in"=w1149, "Report"=w1148) -> ("error out"=w1147:errorcluster, "Pres?"=w1138:bool)  [unwired: 5 in, 2 out]
                  n431 = Increment(x=w1143) -> (x+1=w1140:i32)
                  n432 = Select(t="Pass" ("String"), s=w1138, f="Clog" ("String")) -> (s? t:f=w1139:string)
                  n433 = call "Update 1 Cart Status.vi"("Selection"=Update_Single_Cart."Cart Reagent", "FP"=w1145, "error in (no error)"=w1147, "String"=w1139, "Cartridge"=w1140) -> ("error out"=w1146:errorcluster)  [unwired: 6 in]
                }
              }
            }
          }
          frame "Finish" {
            n434 = Unbundle By Name(w1163) -> ("Config"=w1169:refnum<vi>)
            n435 = Unbundle By Name(w1163) -> ("Start TW"=w1178:refnum<vi>)
            n436 = property class="Clust (strict)"(reference=w1169) -> ("Value"=w1168:T2)  [unwired: 1 in, 2 out]
            n437 = Unbundle By Name(w1168) -> ("Bottom Position"=w1167:dbl)
            n438 = Unbundle By Name(w1163) -> ("Main Clean Cart"=w1164:refnum<vi>)
            n439 = property class="Bool (strict)"(reference=w1178, "Value"=FALSE) -> ()  [unwired: 1 in, 2 out]
            n440 = property class="Bool (strict)"(reference=w1164, "Value"=FALSE, "DisabledEnum"=T13."Enabled" ("Disabled")) -> ()  [unwired: 1 in, 2 out]
            n441 = call "Zaber Manager.vi"("Action"=Mot_Stage_Mngr."Abs Move", "Value"=w1167, "error in (no error)"=w1180) -> ("error out"=w1161:errorcluster)  [unwired: 6 in, 6 out]
            n442 = call "DAQ Manager.vi"("DAQ Mngr Action"=DAQ_Mngr."Pinch Valve Disengage", "error in (no error)"=w1161) -> ("error out"=w1160:errorcluster)  [unwired: 6 in, 7 out]
            n443 = call "Update Cart Status.vi"("Selection"=status_update."Cartridge", "error in (no error)"=w1160, "String"="Finished", "Array"=w1181, "FP"=w1163) -> ("error out"=w1173:errorcluster)  [unwired: 6 in]
            n444 = call "Update Cart Status.vi"("Selection"=status_update."Main Status", "error in (no error)"=w1173, "String"="Thermal Wash is finished, please remove catridges" ("Current Status"), "FP"=w1163) -> ("error out"=w1172:errorcluster)  [unwired: 7 in]
          }
          frame "-rinse wells" {
            n445 = call "Update Cart Status.vi"("Selection"=status_update."Main Status", "error in (no error)"=w1198, "String"="Draining All Wells and Lines", "FP"=w1191) -> ("error out"=w1197:errorcluster)  [unwired: 7 in]
            n446 = Unbundle By Name(w1191) -> ("Config"=w1204:refnum<vi>)
            n447 = property class="Clust (strict)"(reference=w1204) -> ("Value"=w1203:T2)  [unwired: 1 in, 2 out]
            n448 = Unbundle By Name(w1203) -> ("Load Position"=w1202:dbl)
            n449 = call "Zaber Manager.vi"("Action"=Mot_Stage_Mngr."Abs Move", "Value"=w1202, "error in (no error)"=w1197) -> ("error out"=w1201:errorcluster)  [unwired: 6 in, 6 out]
            n450 = call "Run Script.vi"("Script Name"="Drain All Wells", "Main References"=w1191, "error in (no error)"=w1201) -> ("error out"=w1192:errorcluster)  [unwired: 8 in]
            n451 = for {
              N: w1193 -> [w1214]
              shift-right: [w1217] -> w1190
              shift-left: w1192 -> [w1213]
              tunnel: w1191 -> [w1211]
              tunnel: w1191 -> [w1210]
              i -> [w1216]
              n452 = Format Into String(format string="Rinse %d of %d", w1216, w1214) -> (resulting string=w1212:string)  [unwired: 2 in, 1 out]
              n453 = call "Update Cart Status.vi"("Selection"=status_update."Main Status", "error in (no error)"=w1213, "String"=w1212, "FP"=w1211) -> ("error out"=w1218:errorcluster)  [unwired: 7 in]
              n454 = call "Run Script.vi"("Script Name"="Rinse All Wells", "Main References"=w1210, "error in (no error)"=w1218) -> ("error out"=w1217:errorcluster)  [unwired: 8 in]
            }
            n455 = Select(t=Process_Turbo."Error" ("State In 2"), s=w1190, f=Process_Turbo."Idle" ("State In 2")) -> (s? t:f=w1208:T1)
          }
          frame "-fill well" {
            # "Move to TW position if we are not doing liquid check"
            n456 = Unbundle By Name(w1236) -> ("Commands"=w1235:refnum<vi>)
            n457 = property class="Clust (strict)"(reference=w1235) -> ("Value"=w1234:T31)  [unwired: 1 in, 2 out]
            n458 = Unbundle By Name(w1234) -> ("Well #"=w1226:T32, "Bottle #"=w1227:T21)
            n459 = Format Into String(format string="Filling %s with %s", w1226, w1227) -> (resulting string=w1228:string)  [unwired: 2 in, 1 out]
            n460 = call "Update Cart Status.vi"("Selection"=status_update."Main Status", "error in (no error)"=w1233, "String"=w1228, "FP"=w1236) -> ("error out"=w1231:errorcluster)  [unwired: 7 in]
            n461 = call "Run Script.vi"("Script Name"="Fill Well_X Reagent_X" ("name or relative path"), "Main References"=w1236, "error in (no error)"=w1231, "Well X"=w1226, "Bottle X"=w1227) -> ("error out"=w1225:errorcluster)  [unwired: 6 in]
            n462 = Select(t=Process_Turbo."PrePresTest" ("State In 2"), s=w1243, f=Process_Turbo."Idle" ("State In 2")) -> (s? t:f=w1242:T1)
            n463 = Select(t=Process_Turbo."Error" ("State In 2"), s=w1225, f=w1242) -> (s? t:f=w1241:T1)
          }
          frame "-drain all" {
            # "Move to TW position if we are not doing liquid check"
            n464 = Unbundle By Name(w1259) -> ("Commands"=w1258:refnum<vi>)
            n465 = property class="Clust (strict)"(reference=w1258) -> ("Value"=w1257:T31)  [unwired: 1 in, 2 out]
            n466 = Unbundle By Name(w1257) -> ("Well #"=w1251:T32, "Bottle #"=w1252:T21)
            n467 = call "Update Cart Status.vi"("Selection"=status_update."Main Status", "error in (no error)"=w1256, "String"="Draining all wells" ("format string"), "FP"=w1259) -> ("error out"=w1254:errorcluster)  [unwired: 7 in]
            n468 = call "Run Script.vi"("Script Name"="Drain All Wells" ("name or relative path"), "Main References"=w1259, "error in (no error)"=w1254, "Well X"=w1251, "Bottle X"=w1252) -> ("error out"=w1250:errorcluster)  [unwired: 6 in]
            n469 = Select(t=Process_Turbo."PrePresTest" ("State In 2"), s=w1266, f=Process_Turbo."Idle" ("State In 2")) -> (s? t:f=w1265:T1)
            n470 = Select(t=Process_Turbo."Error" ("State In 2"), s=w1250, f=w1265) -> (s? t:f=w1264:T1)
          }
          frame "-clean cartridge" {
            # "clean time"
            # "TODO:  do all of this with one script\nneed to add Pressure X to script handler"
            n471 = call "Update Cart Status.vi"("Selection"=status_update."Main Status", "error in (no error)"=w1315, "String"="Cleaning cartridge", "FP"=w1286) -> ("error out"=w1284:errorcluster)  [unwired: 7 in]
            n472 = call "DAQ Manager.vi"("DAQ Mngr Action"=DAQ_Mngr."Pinch Valve Engage", "error in (no error)"=w1284) -> ("error out"=w1283:errorcluster)  [unwired: 6 in, 7 out]
            n473 = for {
              shift-right: [w1336] -> w1299
              shift-left: w1283 -> [w1337]
              tunnel: w1286 -> [w1335]
              tunnel: w1270 -> [w1334] mode=indexing
              tunnel: "Drain Well X" ("name or relative path") -> [w1333]
              i -> [w1332]
              n474 = case shown="True" w1334 {
                tunnel: w1337 -> [w1338 w1343]
                tunnel: [w1338 w1341] -> w1336
                tunnel: w1335 -> [_ w1342]
                tunnel: w1333 -> [_ w1340]
                tunnel: w1332 -> [_ w1339]
                frame False {
                }
                frame True {
                  n475 = call "Run Script.vi"("Script Name"=w1340, "Main References"=w1342, "error in (no error)"=w1343, "Drain X"=w1339, "Well X"=w1339) -> ("error out"=w1341:errorcluster)  [unwired: 6 in]
                }
              }
            }
            n476 = Unbundle By Name(w1286) -> ("Commands"=w1313:refnum<vi>)
            n477 = Unbundle By Name(w1286) -> ("Config"=w1305:refnum<vi>)
            n478 = property class="Clust (strict)"(reference=w1305) -> ("Value"=w1304:T2)  [unwired: 1 in, 2 out]
            n479 = Unbundle By Name(w1304) -> ("Bottom Position"=w1277:dbl, "TW Position"=w1291:dbl, "Dry Time(s)"=w1289:dbl)
            n480 = property class="Clust (strict)"(reference=w1313) -> (reference out=w1308:refnum<vi>, "Value"=w1310:T31)  [unwired: 1 in, 1 out]
            n481 = for {
              shift-right: [w1323] -> w1297
              shift-left: w1299 -> [w1324]
              tunnel: w1286 -> [w1322]
              tunnel: w1270 -> [w1321] mode=indexing
              tunnel: "Fill Well_X Reagent_X" ("name or relative path") -> [w1320]
              i -> [w1319]
              n482 = case shown="True" w1321 {
                tunnel: w1324 -> [w1325 w1331]
                tunnel: [w1325 w1329] -> w1323
                tunnel: w1322 -> [_ w1330]
                tunnel: w1320 -> [_ w1328]
                tunnel: w1319 -> [_ w1327]
                frame False {
                }
                frame True {
                  n483 = call "Run Script.vi"("Script Name"=w1328, "Main References"=w1330, "error in (no error)"=w1331, "Drain X"=w1327, "Well X"=w1327, "Bottle X"=Bottles."H2O") -> ("error out"=w1329:errorcluster)  [unwired: 5 in]
                }
              }
            }
            n484 = call "Zaber Manager.vi"("Action"=Mot_Stage_Mngr."Abs Move", "Value"=w1291, "error in (no error)"=w1297) -> ("error out"=w1295:errorcluster)  [unwired: 6 in, 6 out]
            n485 = Bundle By Name(cluster=w1310, "Clean&Dry Cartridge"=FALSE ("Check for leaks")) -> (w1307:T31)
            n486 = call "16CH Denkovi Manager.vi"("Action"=16CH_Denkovi_Mngr."Pres ON", "error in (no error)"=w1295, "Relays In"=w1270) -> ("error out"=w1292:errorcluster)  [unwired: 6 in, 2 out]
            n487 = call "Delay with Cancel 2.vi"("Insert Error"=FALSE, "error in (no error)"=w1292, "Delay(s)"=180.0) -> ("error out"=w1280:errorcluster)  [unwired: 7 in, 1 out]
            n488 = for {
              shift-right: [w1348] -> w1273
              shift-left: w1280 -> [w1349]
              tunnel: w1286 -> [w1347]
              tunnel: w1270 -> [w1346] mode=indexing
              tunnel: "Drain Well X" ("name or relative path") -> [w1345]
              i -> [w1344]
              n489 = case shown="True" w1346 {
                tunnel: w1349 -> [w1350 w1355]
                tunnel: [w1350 w1353] -> w1348
                tunnel: w1347 -> [_ w1354]
                tunnel: w1345 -> [_ w1352]
                tunnel: w1344 -> [_ w1351]
                frame False {
                }
                frame True {
                  n490 = call "Run Script.vi"("Script Name"=w1352, "Main References"=w1354, "error in (no error)"=w1355, "Drain X"=w1351, "Well X"=w1351) -> ("error out"=w1353:errorcluster)  [unwired: 6 in]
                }
              }
            }
            n491 = call "16CH Denkovi Manager.vi"("Action"=16CH_Denkovi_Mngr."Pres ON", "error in (no error)"=w1273, "Relays In"=w1270) -> ("error out"=w1272:errorcluster)  [unwired: 6 in, 2 out]
            n492 = call "Delay with Cancel 2.vi"("Insert Error"=FALSE, "error in (no error)"=w1272, "Delay(s)"=w1289) -> ("error out"=w1276:errorcluster)  [unwired: 7 in, 1 out]
            n493 = call "DAQ Manager.vi"("DAQ Mngr Action"=DAQ_Mngr."Pinch Valve Disengage", "error in (no error)"=w1276) -> ("error out"=w1274:errorcluster)  [unwired: 6 in, 7 out]
            n494 = call "16CH Denkovi Manager.vi"("Action"=16CH_Denkovi_Mngr."Pres Vent&Close", "error in (no error)"=w1274, "Relays In"=w1270) -> ("error out"=w1275:errorcluster)  [unwired: 6 in, 2 out]
            n495 = call "Zaber Manager.vi"("Action"=Mot_Stage_Mngr."Abs Move", "Value"=w1277, "error in (no error)"=w1275) -> ("error out"=w1279:errorcluster)  [unwired: 6 in, 6 out]
            n496 = property class="Clust (strict)"(reference=w1308, error in=w1279, "Value"=w1307) -> (error out=w1303:errorcluster)  [unwired: 1 out]
            n497 = Select(t=Process_Turbo."Error" ("State In 2"), s=w1303, f=Process_Turbo."Idle" ("State In 2")) -> (s? t:f=w1318:T1)
          }
          frame "-check cartridge" {
            n498 = call "Update Cart Status.vi"("Selection"=status_update."Main Status", "error in (no error)"=w1388, "String"="Checking cartridge", "FP"=w1376) -> ("error out"=w1363:errorcluster)  [unwired: 7 in]
            n499 = call "DAQ Manager.vi"("DAQ Mngr Action"=DAQ_Mngr."Pinch Valve Engage", "error in (no error)"=w1363) -> ("error out"=w1362:errorcluster)  [unwired: 6 in, 7 out]
            n500 = Unbundle By Name(w1376) -> ("Commands"=w1386:refnum<vi>)
            n501 = disable-structure shown="Enabled" {
              disable-tunnel: [w1411 w1426] -> w1383
              disable-tunnel: w1376 -> [w1410 _]
              disable-tunnel: w1366 -> [w1409 _]
              disable-tunnel: w1362 -> [w1408 w1426]
              frame Disabled {
                n502 = for {
                  shift-right: [w1415] -> w1411
                  shift-left: w1408 -> [w1416]
                  tunnel: w1410 -> [w1414]
                  tunnel: w1409 -> [w1413] mode=indexing
                  i -> [w1412]
                  n503 = case shown="True" w1413 {
                    tunnel: w1416 -> [w1417 w1423]
                    tunnel: [w1417 w1421] -> w1415
                    tunnel: w1414 -> [_ w1420]
                    tunnel: w1412 -> [_ w1418]
                    frame False {
                    }
                    frame True {
                      n504 = call "Run Script.vi"("Script Name"="Drain Well X" ("name or relative path"), "Main References"=w1420, "error in (no error)"=w1423, "Drain X"=w1418, "Well X"=w1418) -> ("error out"=w1422:errorcluster)  [unwired: 6 in]
                      n505 = call "Run Script.vi"("Script Name"="Fill Well_X Reagent_X" ("name or relative path"), "Main References"=w1420, "error in (no error)"=w1422, "Drain X"=w1418, "Well X"=w1418, "Bottle X"=Bottles."H2O") -> ("error out"=w1421:errorcluster)  [unwired: 5 in]
                    }
                  }
                }
              }
              frame Enabled {
              }
            }
            n506 = Unbundle By Name(w1376) -> ("Config"=w1375:refnum<vi>)
            n507 = property class="Clust (strict)"(reference=w1375) -> ("Value"=w1374:T2)  [unwired: 1 in, 2 out]
            n508 = property class="Clust (strict)"(reference=w1386) -> (reference out=w1380:refnum<vi>, "Value"=w1382:T31)  [unwired: 1 in, 1 out]
            n509 = Unbundle By Name(w1374) -> ("Bottom Position"=w1373:dbl)
            n510 = call "Detect Transition to TW.vi"("Main References"=w1376, "error in (no error)"=w1383, "Cart Array"=w1366) -> ("error out"=w1368:errorcluster, "Analysis"=w1369:T7[])  [unwired: 7 in]
            n511 = call "16CH Denkovi Manager.vi"("Action"=16CH_Denkovi_Mngr."Pres Vent&Close", "error in (no error)"=w1368, "Relays In"=w1366) -> ("error out"=w1367:errorcluster)  [unwired: 6 in, 2 out]
            n512 = Bundle By Name(cluster=w1382, "Check for leaks"=FALSE, "Cart Test Array"=w1369) -> (w1379:T31)
            n513 = call "Zaber Manager.vi"("Action"=Mot_Stage_Mngr."Abs Move", "Value"=w1373, "error in (no error)"=w1367) -> ("error out"=w1360:errorcluster)  [unwired: 6 in, 6 out]
            n514 = call "DAQ Manager.vi"("DAQ Mngr Action"=DAQ_Mngr."Pinch Valve Disengage", "error in (no error)"=w1360) -> ("error out"=w1359:errorcluster)  [unwired: 6 in, 7 out]
            n515 = disable-structure shown="Enabled" {
              disable-tunnel: w1359 -> [w1395 w1407]
              disable-tunnel: w1376 -> [w1394 _]
              disable-tunnel: [w1393 w1407] -> w1372
              disable-tunnel: w1366 -> [w1392 _]
              frame Disabled {
                n516 = for {
                  shift-right: [w1399] -> w1393
                  shift-left: w1395 -> [w1400]
                  tunnel: w1394 -> [w1398]
                  tunnel: w1392 -> [w1397] mode=indexing
                  i -> [w1396]
                  n517 = case shown="True" w1397 {
                    tunnel: w1400 -> [w1401 w1405]
                    tunnel: [w1401 w1403] -> w1399
                    tunnel: w1398 -> [_ w1404]
                    tunnel: w1396 -> [_ w1402]
                    frame False {
                    }
                    frame True {
                      n518 = call "Run Script.vi"("Script Name"="Drain Well X" ("name or relative path"), "Main References"=w1404, "error in (no error)"=w1405, "Drain X"=w1402, "Well X"=w1402) -> ("error out"=w1403:errorcluster)  [unwired: 6 in]
                    }
                  }
                }
              }
              frame Enabled {
              }
            }
            n519 = property class="Clust (strict)"(reference=w1380, error in=w1372, "Value"=w1379) -> (error out=w1371:errorcluster)  [unwired: 1 out]
            n520 = Select(t=Process_Turbo."Idle" ("State In 2"), s=w1371, f=Process_Turbo."Idle" ("State In 2")) -> (s? t:f=w1391:T1)
          }
        }
      }
    }
    frame Error {
      (unwired) T34 {"negative limit switch"=FALSE, "positive limit switch"=FALSE, "home switch"=FALSE, "position marker"=FALSE, "device enable"=FALSE, "quick stop"=FALSE, "general purpose J"=FALSE, "general purpose I"=FALSE, "general purpose H"=FALSE, "general purpose G"=FALSE, "general purpose F"=FALSE, "general purpose E"=FALSE, "general purpose D"=FALSE, "general purpose C"=FALSE, "general purpose B"=FALSE, "general purpose A"=FALSE} ("digital inputs")
    }
  }
  "error out" <- w11
  "Wash Array" <- w8
  "Reports" <- w6
  "State Out" <- w2
